vi "HostoldMain.vi"() -> ()   [LabVIEW 2009]
uses:
  <vilib>/rvi/interface/nirviOpenFPGA/nirviOpenFPGA.xnode
  <vilib>/rvi/interface/nirviReadWriteControl/nirviReadWriteControl.xnode
  <vilib>/rvi/interface/nirviCloseFPGA/nirviCloseFPGA.xnode
  States.ctl
  <vilib>/rvi/interface/nirviMethod/nirviMethod.xnode
  Pulse Acquisition/5122-States.ctl
  <instrlib>/niScope/Configure/Trigger/niScope Configure Trigger Edge.vi
  <instrlib>/niScope/Acquire/Fetch/niScope Fetch.vi
  <vilib>/Analysis/NI_AALPro.lvlib
  <vilib>/Utility/file.llb/Write To Spreadsheet File (DBL).vi
  B Field control Signal/B-Generator States.ctl
  <vilib>/DAQmx/create/channels.llb/DAQmx Create Channel (AO-Voltage-Basic).vi
  <vilib>/DAQmx/configure/timing.llb/DAQmx Timing (Sample Clock).vi
  <vilib>/DAQmx/configure/trigger.llb/DAQmx Start Trigger (Digital Edge).vi
  Program Files (x86)/National Instruments/LabVIEW 2009/resource/objmgr/daqmx.rc
  <vilib>/DAQmx/write.llb/DAQmx Write (Analog 1D DBL 1Chan NSamp).vi
  <vilib>/Utility/error.llb/DialogType.ctl
  FPGA Bitfiles/MOT2.lvproj_FPGA Target_FPGAvi.vi.lvbitx
  Signal Options.ctl
  FPGAvi.vi
  Sequence.ctl
  <instrlib>/Agilent ESG Series/Agilent ESG Series.lvlib
  Raman Measure/Raman.ctl
  <vilib>/DAQmx/create/channels.llb/DAQmx Create Channel (AI-Voltage-Basic).vi
  <vilib>/DAQmx/read.llb/DAQmx Read.vi
  <vilib>/DAQmx/read.llb/DAQmx Read (Analog 2D DBL NChan NSamp).vi
  <vilib>/Analysis/NI_AALBase.lvlib
  <vilib>/userDefined/High Color/nirio_resource_hc.ctl
  <instrlib>/niScope/Controls/niScope vertical coupling.ctl
panel:
  out "data":dbl[][](array[numeric]) format="%0.6f"
  in  "Output  Trigger Sign (DIO1)":bool
  in  "Signal Trigger Source (DIO0)":bool=TRUE
  in  "Pulse Selection":bool
  in  "Switch Chopper \nWindow Trigger":bool
  in  "Master Stop":bool
  in  "Tab Control":T1(tab)
  out "Acquisition Rate":dbl[unit]=0.02 min=0.0 max=107374.18239999999
  in  "Pulse Repetition Period":dbl[unit]=0.02
  out "Memory Sequence Duration":dbl[unit]=0.02 min=0.0 max=107374.18239999999
  out "Chopper 1/2 Dark Time":dbl[unit]
  in  "DLCZ Period":dbl[unit]=1e-06
  in  "DLCZ Pulse Duration":dbl[unit]=5.0000000000000004e-08
  in  "DLCZ Stop":dbl[unit]=0.004 caption="Stop"
  in  "DLCZ Start":dbl[unit] caption="Start"
  in  "B-Field Extinction Time":dbl[unit]=0.00125 min=0.0 max=107374.18239999999
  in  "Min. Measurement Period":dbl[unit]=0.02 caption="Meas. Period" min=0.0 max=107374.18239999999
  in  "Opt Density Delay (DIO7)":dbl[unit]
  in  "Opt Density Duration (DIO7)":dbl[unit]=0.000125
  in  "Signal Delay (DIO6)":dbl[unit]
  in  "Signal Duration (DIO6)":dbl[unit]=0.000125
  in  "Control Delay(DIO5/1)":dbl[unit] min=0.0 max=107374.18239999999
  in  "Control Duration (DIO5/1)":dbl[unit]=0.000125 min=0.0 max=107374.18239999999
  in  "FPGA Target":T2="FPGA"
  out "Active":bool
  in  "Memory Mode":T3=enum."Generate DLCZ Pulses"
  in  "Trapping (DIO3)":dbl[unit]=0.0015 min=0.0 max=107374.18239999999
  in  "Repump (DIO4)":dbl[unit]=0.0015
  in  "Pump (DIO8)":dbl[unit]=0.0015
  out "Graphing":bool
  out "Generated Signals":digitalwaveform(graph)
  in  "Activate Raman Acquisition":bool=TRUE
  in  "Scan Frequency":bool
  out "Acquisition Count":i32
  in  "Number of Measurements":u32=10
  in  "Samples per Channel":i32=2048 caption="Measurement Samples"
  in  "VISA session":refnum<visa-resource-name>="GPIB0::19::INSTR"
  out "Current Frequency":dbl[unit]
  in  "Start Frequency":dbl[unit]=-5000000.0
  in  "Stop Frequency":dbl[unit]=5000000.0
  in  "Resonance Frequency":dbl[unit]=100000000.0
  in  "Upper Threshold (% of Max)":dbl=80.0
  in  "Lower Threshold (% of Min)":dbl=120.0
  in  "Number of Frequency Intervals":u32=100
  out "Frequency Interval":dbl[unit]
  in  "Raman Measurement File":path=path "C:/Users/atomes/Desktop/Labview Projects/MOT2/raman.txt"
  out "Measurement":dbl[][](graph) caption="Pulse Monitor"
  out "Raman Measure":cluster{dbl[], dbl[]}[](graph)
  in  "Ramand Control Duration (DIO5)":dbl[unit]=0.000125 min=0.0 max=107374.18239999999
  in  "Raman Control Delay(DIO5)":dbl[unit] min=0.0 max=107374.18239999999
  in  "Raman Signal Delay (DIO6)":dbl[unit]
  in  "Raman Signal Duration (DIO6)":dbl[unit]=0.000125
  in  "Acquisition Delay":dbl[unit] format="%.2f"
  out "Interval Between Samples":dbl[unit]
  out "Actual Sample Rate":dbl[unit]
  in  "Desired Sample Rate":dbl[unit]=100000000.0 caption="Min. Sample Rate" step=1.0 format="%.2p"
  in  "Acquisition Time per Pulse":dbl[unit]=0.0005 format="%#.2g"
  out "Acquisitions Remaining":i32 caption="Number of Runs"
  in  "Data Output":path=path "F:/data/test.txt"
  in  "Number of Pulses to Record":i32=1 caption="Number of Runs" format="%.0p"
  out "Total Acquired Time":dbl[unit]
  out "Total Number of Datapoints":i32=1000000
  out "Total Experiment Time":dbl[unit]
  out "Number of Samples per Pulse":i32
  in  "Vertical range (0 to 10V)":dbl[unit]=4.0 caption="Vertical Range (V)" format="%.2f"
  in  "Vertical coupling":T4=1 caption="Vertical Coupling" items=["AC", "DC", "Ground"]
  in  "Channel":u16(ring) items=["0", "1"]
  out "Acquisition Sequence":dbl[][](graph)
  in  "Get Reference Parameters":bool
  in  "Capture":bool
  in  "Acquire Data":bool
  out "Global EIT Delay":dbl[unit] format="%#.2g"
  out "Risetime Chart":cluster{dbl}(graph)
  out "Falltime Chart":cluster{dbl}(graph)
  out "Width Chart":cluster{dbl}(graph)
  out "Delay Chart":cluster{dbl}(graph)
  out "Amplitude Chart":cluster{dbl}(graph)
  out "Risetime":string
  out "Falltime":string
  out "Pulse Width":string
  out "Delay":string
  out "Amplitude":string
  out "Memory Duration":dbl[unit]
  in  "Global Delay":dbl[unit]=3e-06
  in  "High Voltage (V Hi)":dbl[unit]=5.0
  in  "Trigger Control":bool=TRUE
  in  "Activate B-Field":bool=TRUE
  out "B-Field Control Signal":dbl[](graph)
  in  "V4":dbl[unit]
  in  "V3":dbl[unit]
  in  "V2":dbl[unit]=-5.0
  in  "V1":dbl[unit]=-5.0 min=-10.0 max=10.0
  in  "B":dbl[unit]=0.003
  in  "A":dbl[unit]=9.999999999999999e-05
  out "t_last_chop+t_dark-t_off":dbl[unit]
  out "Current State":T5
  out "Cut Initiated":dbl[unit]
  out "B-Field Extinction Time 2":dbl[unit]
  out "Memory Mode 2":T3=enum."Coherent Memory Sequence"
  in  "Epsilon":dbl[unit]
  out "Memory Timer":dbl[unit]
  out "Global Time":dbl[unit]
  out "t_chop":dbl[unit]
  out "T_last-chop + t_dark":dbl[unit]
  out "Last DLCZ Period":dbl[unit]
  out "Reference Pulse":dbl[](array[numeric])
  out "Channel String":string
  # "Chopper"
  # "Internal"
  # "All Pulses"
  # "1 out of 2 Pulses"
  # "Delays"
  # "Durations"
  # "Chopper Measurement and MOT Timing"
  # "DLCZ Pulse Train (DIO5)"
  # "Width"
  # "Period"
  # "Optical Density (DIO7)"
  # "Signal (DIO6)"
  # "Control  (DIO5)"
  # "Extinction Time"
  # "Delays"
  # "Durations"
  # "Raman Signal (DIO6)"
  # "Raman Control (DIO5)"
  # "Optical Pulse Acquisition"
  # "Pulse Statistics"
  # "Trigger must be sent \nto begin generation"
  # "Example Diagram"
  # "Voltages"
  # "Intervals"
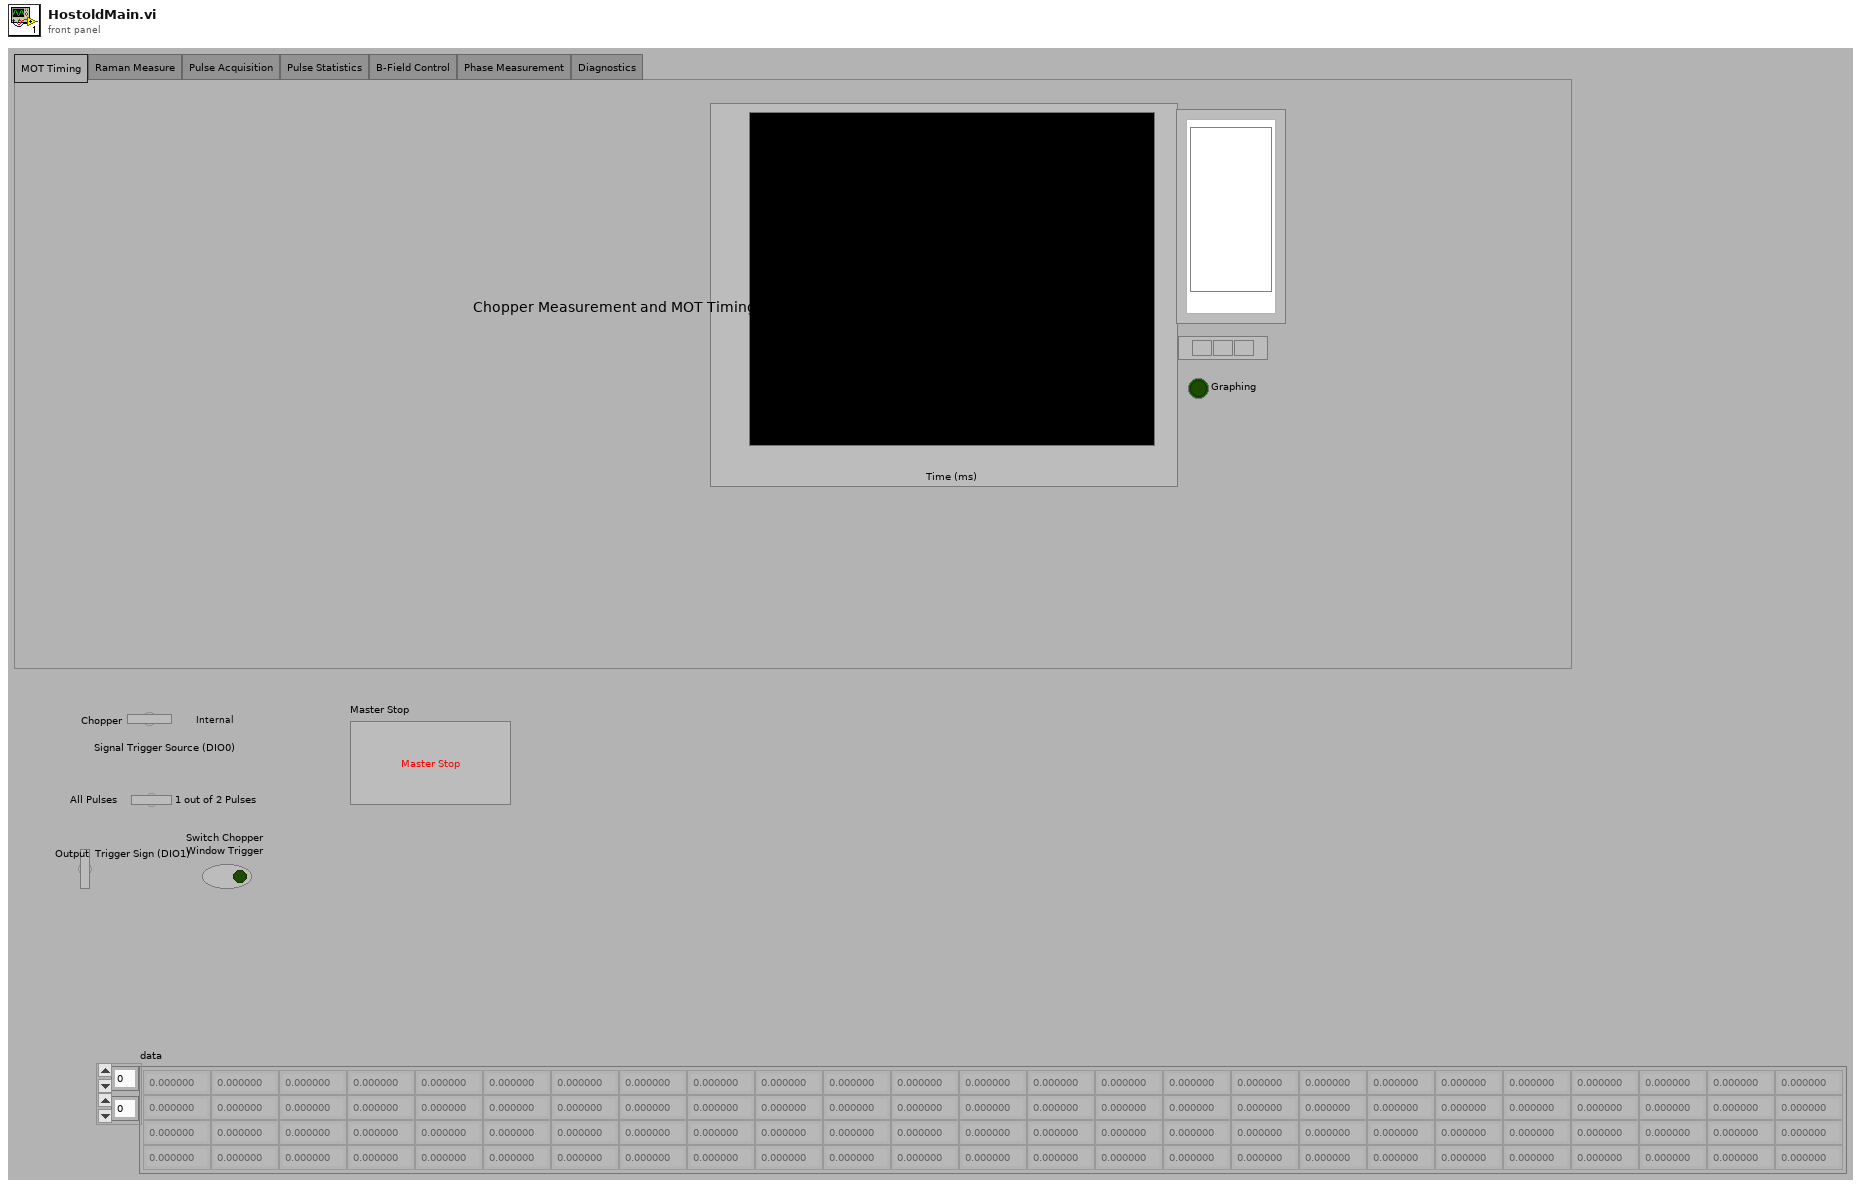
[diagram p1: front panel]
types:
  T1 = enum32{"MOT Timing", "Raman Measure", "Pulse Acquisition", "Pulse Statistics", "B-Field Control", "Phase Measurement", "Diagnostics"}
  T2 = typedef "nirio_resource_hc.ctl" = tag
  T3 = typedef "Signal Options.ctl" = enum16{"Cycle Trap - Standby", "Generate DLCZ Pulses", "Measure Optical Density", "Measure Raman", "Single Photon Memory Efficiency", "Coherent Memory Sequence", "Squeezed AOM Memory Sequence", "Squeezed Chopper Memory Sequence"}
  T4 = typedef "niScope vertical coupling.ctl" = i32
  T5 = typedef "Sequence.ctl" = enum16{"Build MOT", "Memory Sequence", "Alignment - Lights On"}
  T6 = typedef "Raman.ctl" = enum16{"Initialize", "Monitor Pulses", "Stop Raman Acquisition", "Scan Frequency", "Output Data", "Standby"}
  T7 = typedef "States.ctl" = enum16{"Initialize", "Send Data", "Receive Data", "Update Graph", "Check for Activity", "Close"}
  T8 = typedef "DialogType.ctl" = u16
  T9 = typedef "B-Generator States.ctl" = enum16{"Initialize", "Start Task", "Check Task", "Stop Task", "Stop"}
  T10 = typedef "5122-States.ctl" = enum16{"Initialize Card", "Continuous Mode", "Fetch", "Snapshot Acquistion", "Standby", "Record DataFile", "Exit"}
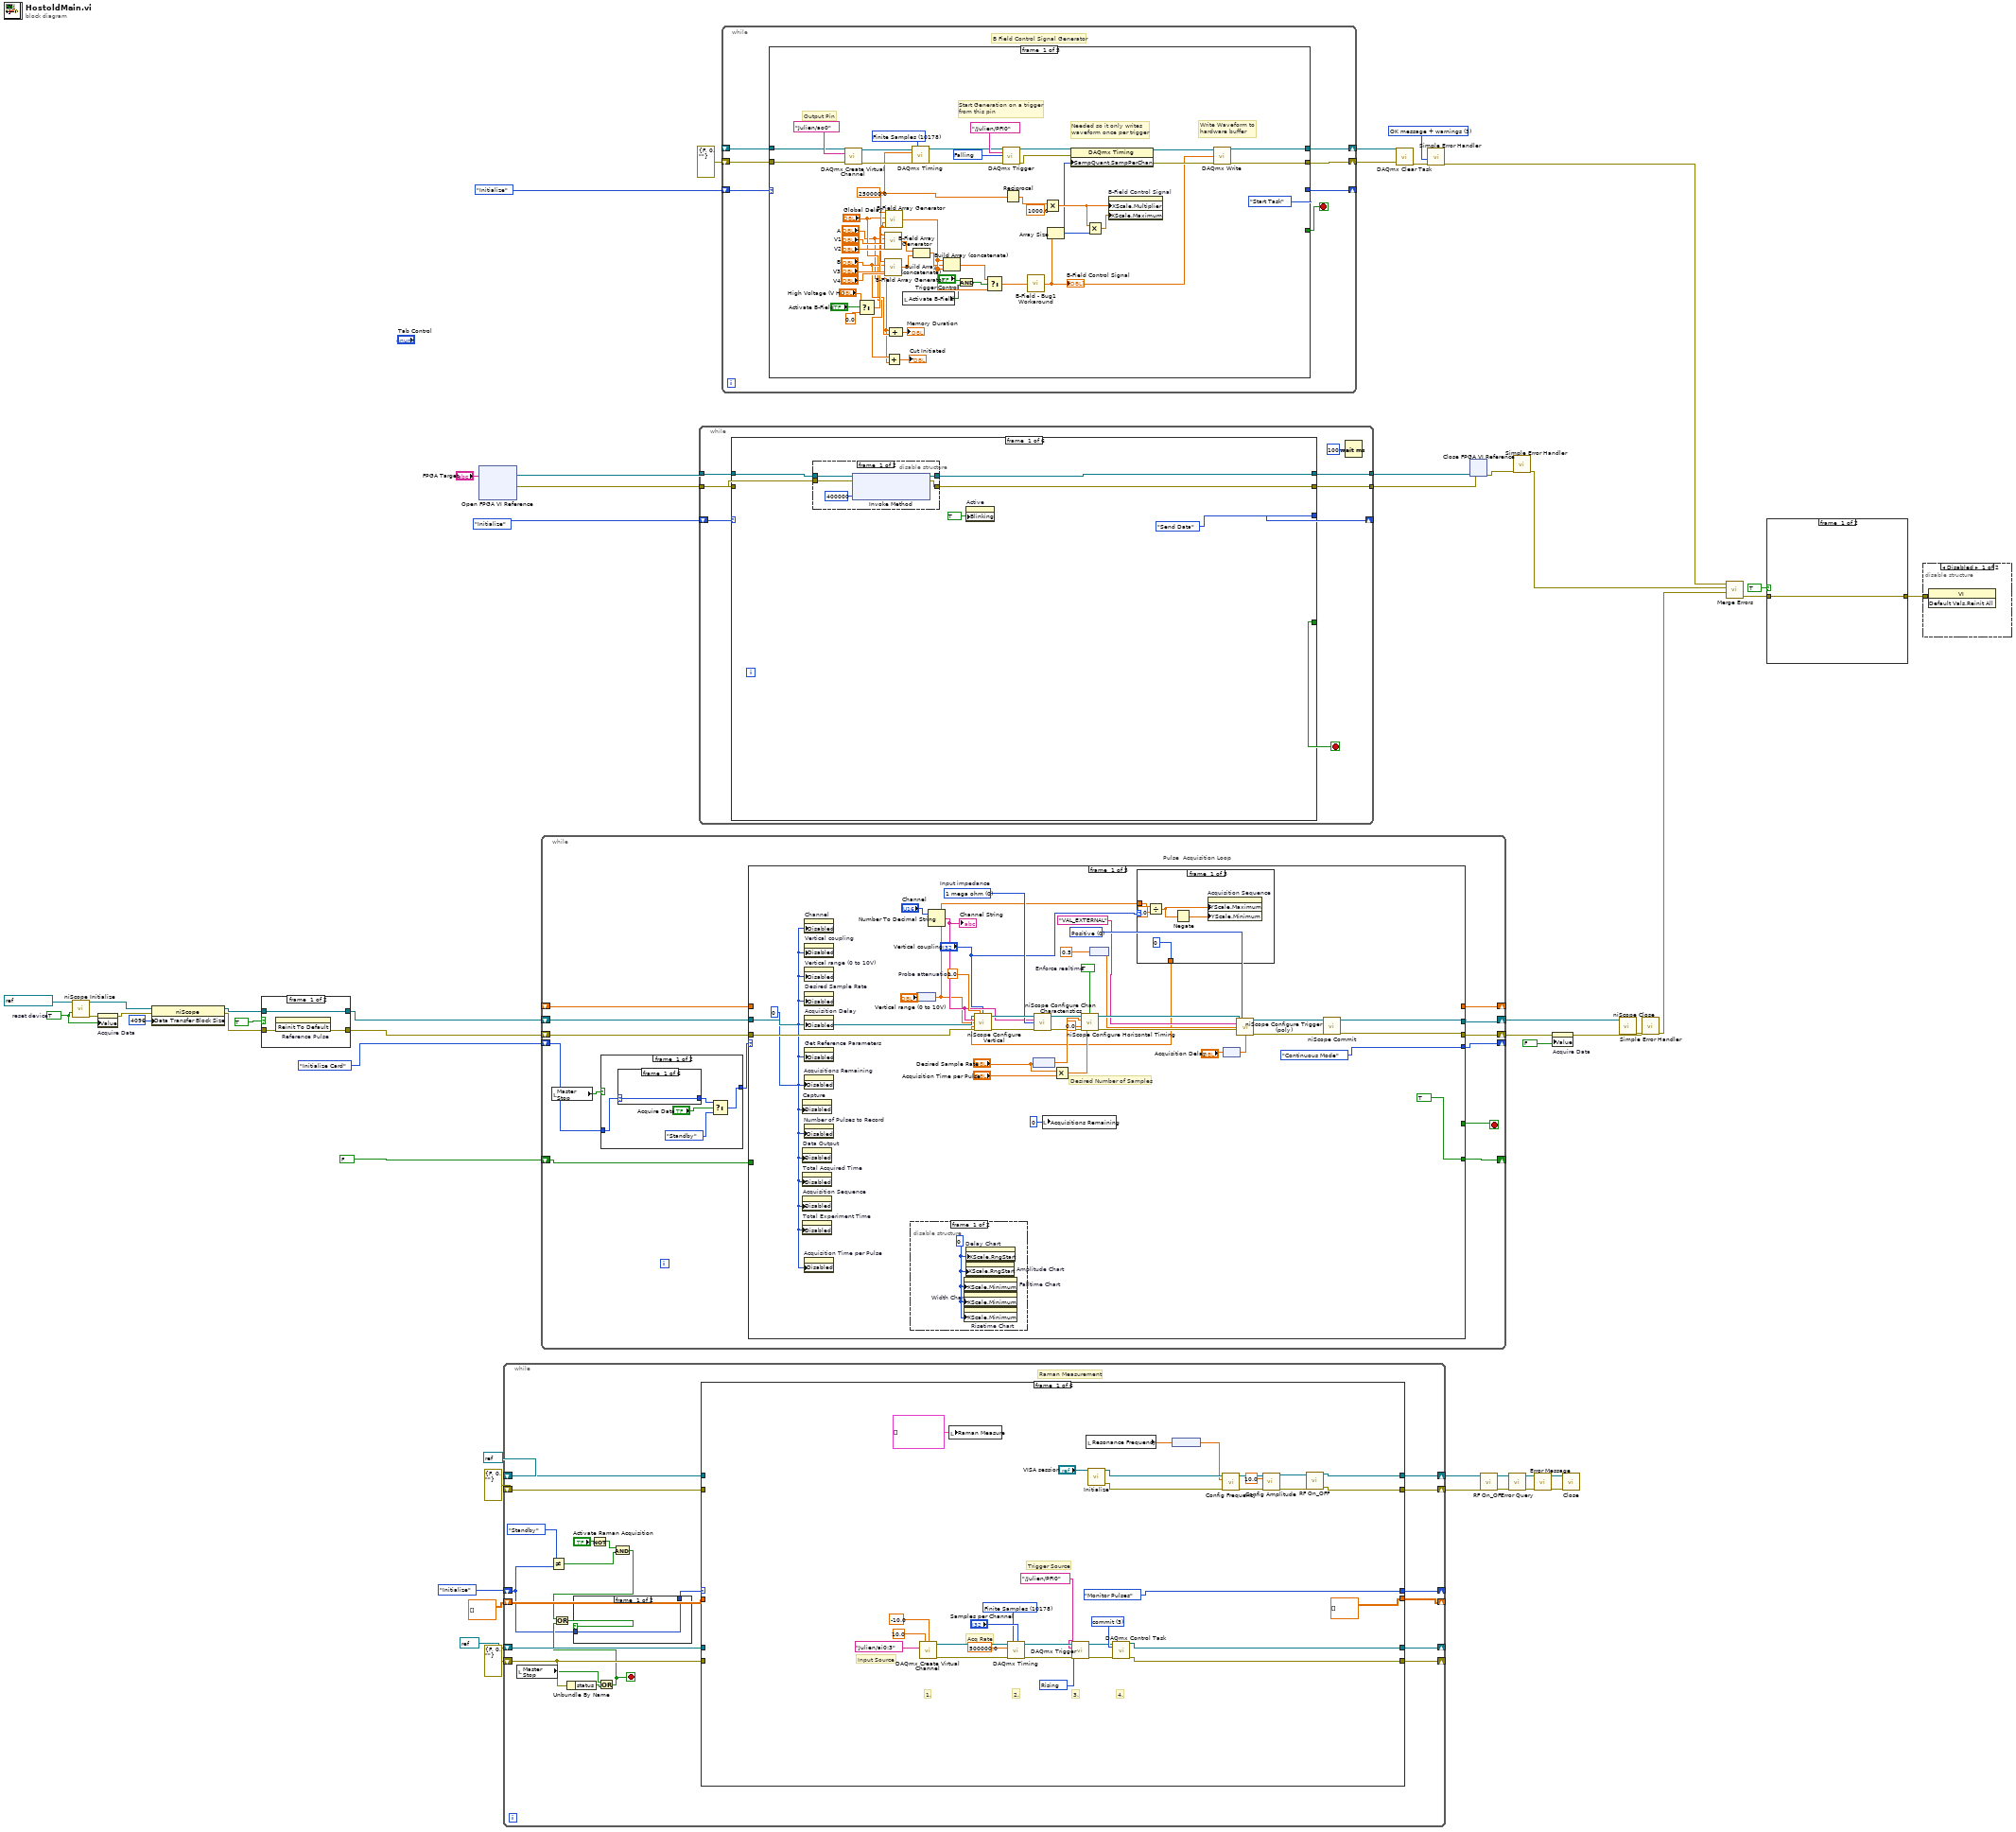
[diagram p0: block diagram]
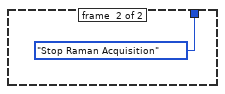
[diagram p2: hidden frame]
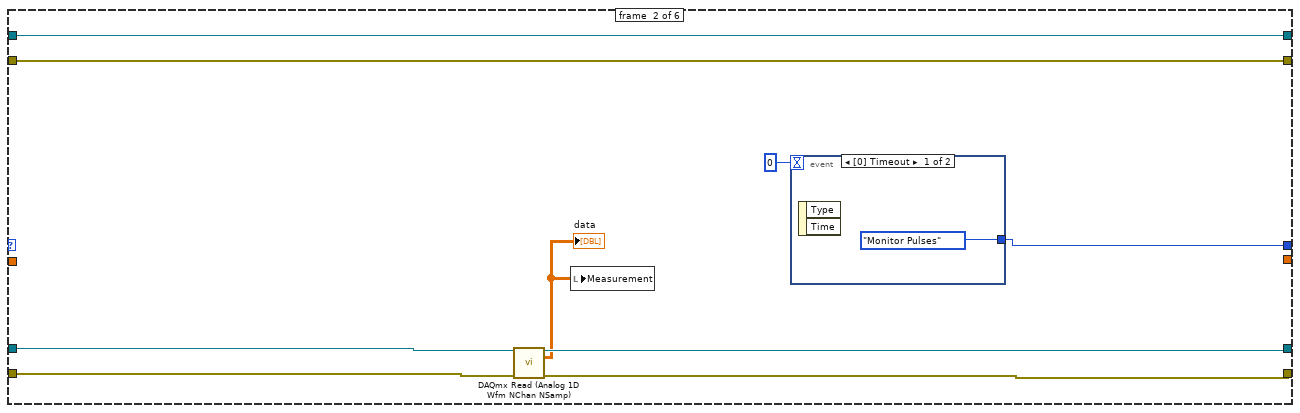
[diagram p3: hidden frame]
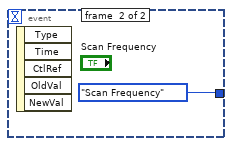
[diagram p4: hidden frame]
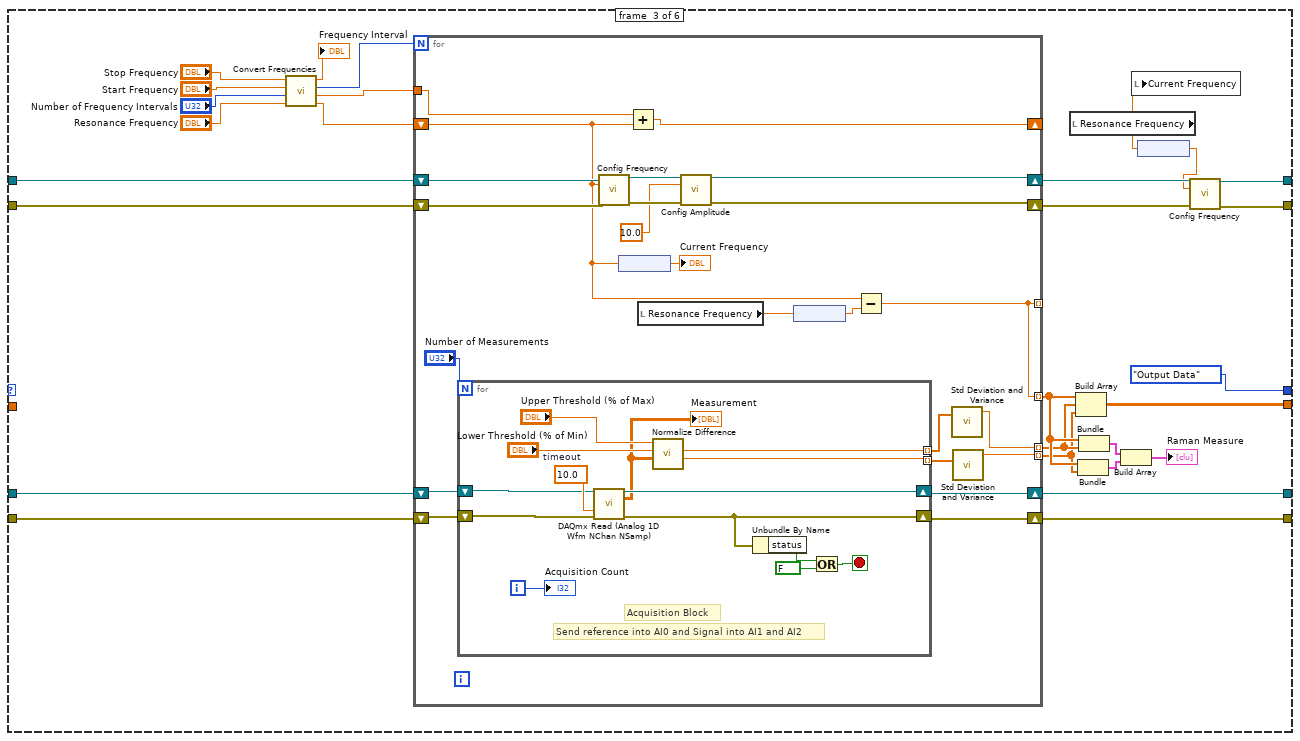
[diagram p5: hidden frame]
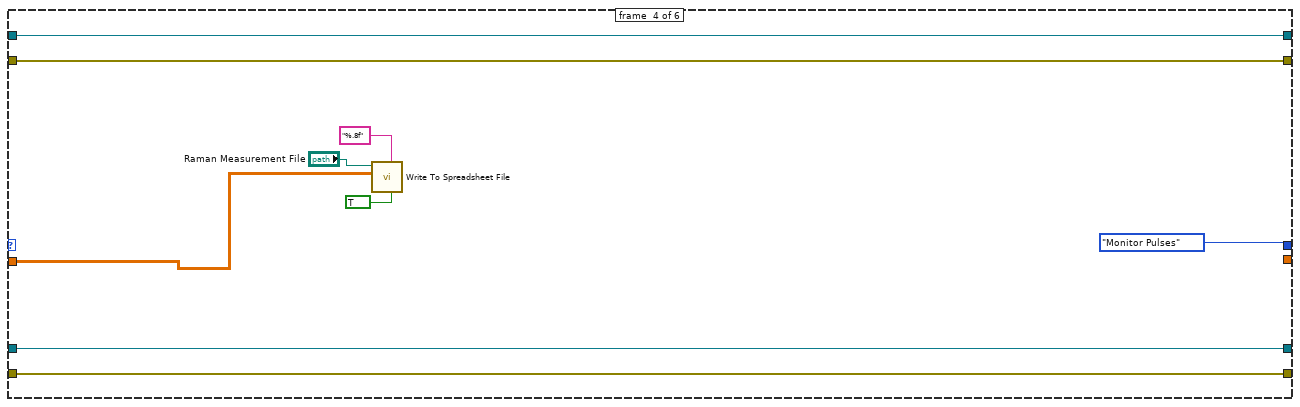
[diagram p6: hidden frame]
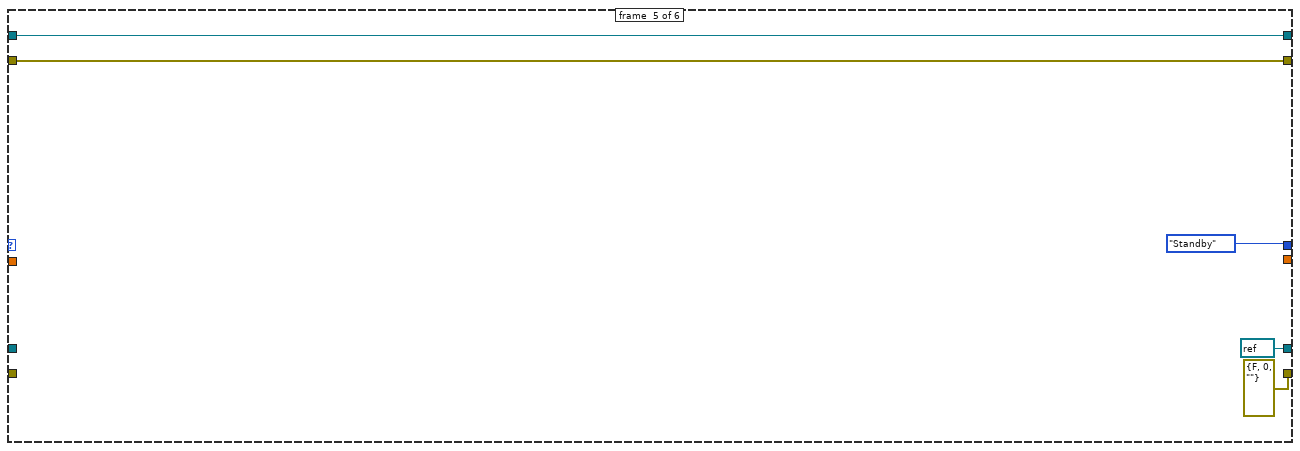
[diagram p7: hidden frame]
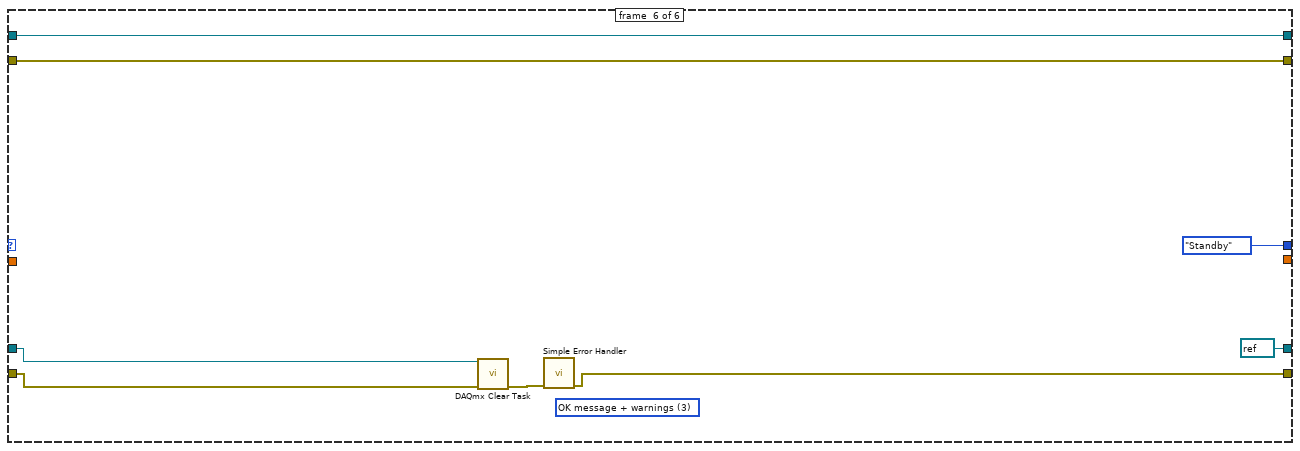
[diagram p8: hidden frame]
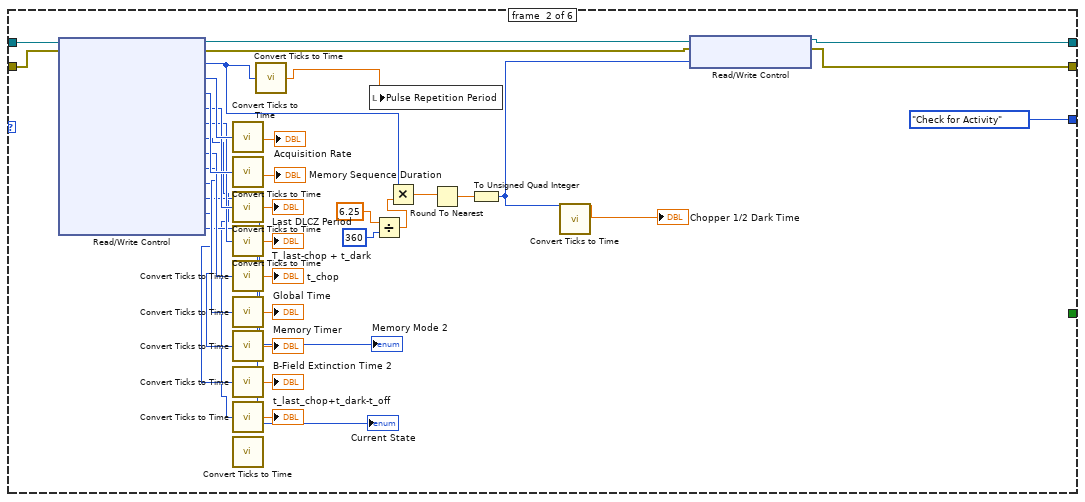
[diagram p10: hidden frame]
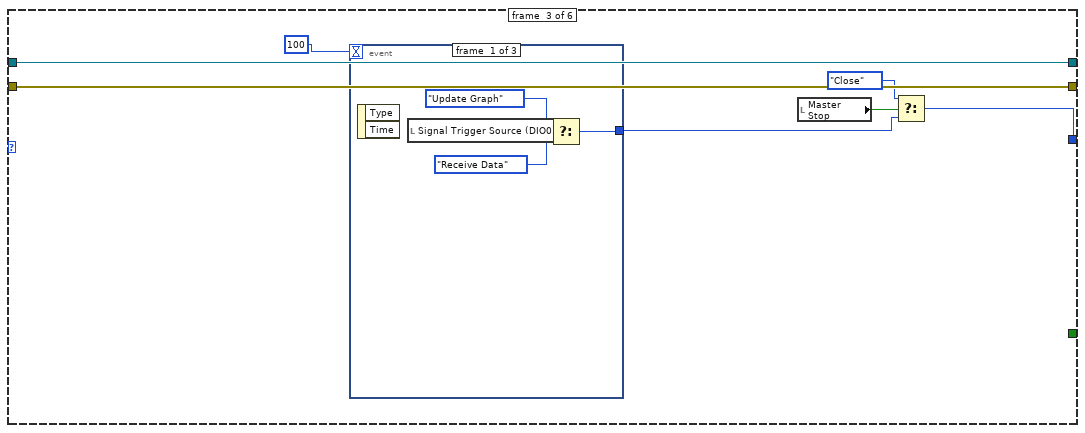
[diagram p11: hidden frame]
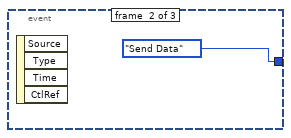
[diagram p12: hidden frame]
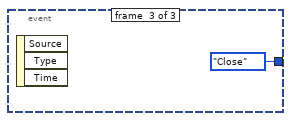
[diagram p13: hidden frame]
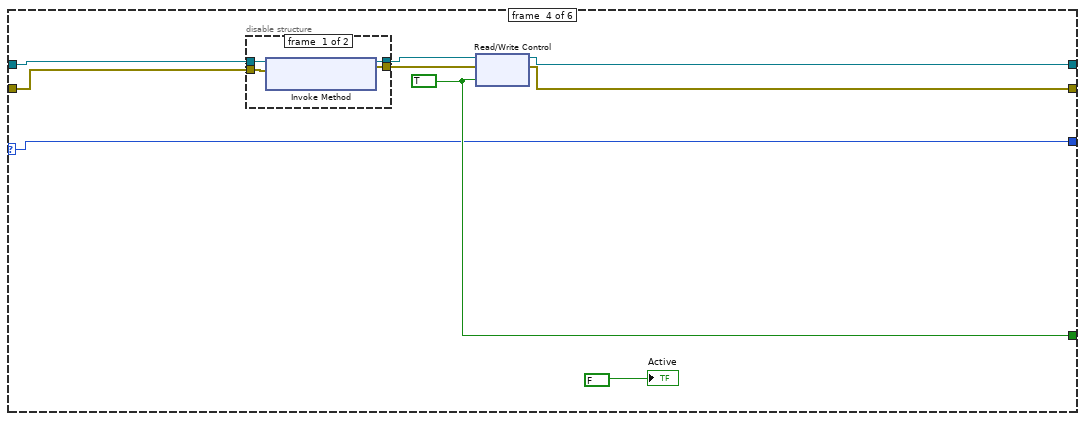
[diagram p14: hidden frame]
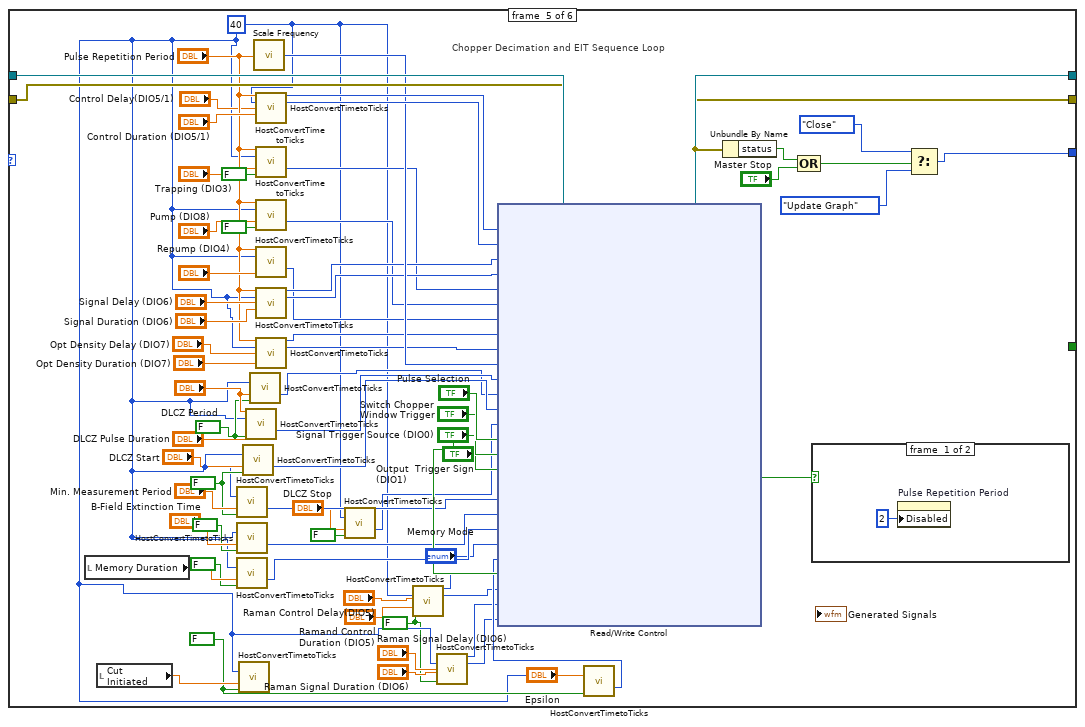
[diagram p16: hidden frame]
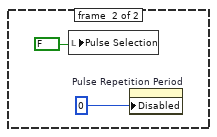
[diagram p17: hidden frame]
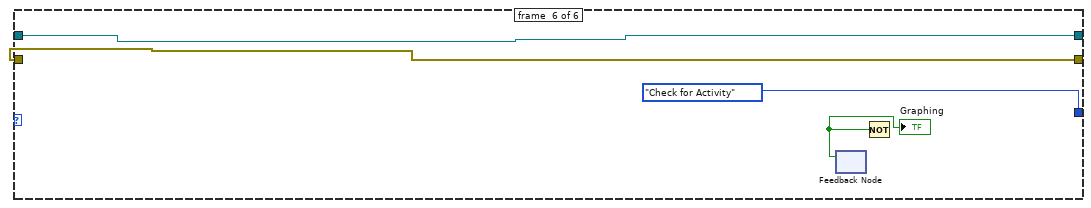
[diagram p18: hidden frame]
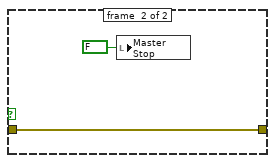
[diagram p20: hidden frame]
diagram:
  w33 = T8 3 items=["no dialog", "OK message", "continue or stop message", "OK message + warnings", "continue/stop + warnings"] ("type of dialog (OK msg:1)")
  w44 = TRUE  # reset device
  n1 = call <instrlib>:"niScope Initialize.vi"("resource name"=refnum<k15> "Acquisition" ("Resource name 5"), "reset device"=w44) -> ("instrument handle"=w48:refnum<k15>, "error out"=w46:errorcluster)  [unwired: 2 in, 10 out]
  n2 = property on="Acquire Data" class="Bool (strict)"(error in=w46, "Value"=w44) -> (error out=w45:errorcluster)  [unwired: 1 in, 1 out]
  n3 = property class="niScope"(reference=w48, error in=w45, "Data Transfer Block Size"=4096) -> (reference out=w38:refnum<k15>, error out=w36:errorcluster)
  n4 = case shown="True" TRUE {
    tunnel: [w53 w55] -> w37
    tunnel: w38 -> [w53 w55]
    tunnel: [w52 w54] -> w35
    tunnel: w36 -> [w52 w54]
    frame #0 {
      n5 = invoke on="Reference Pulse" class="Arr (strict)" method="Reinit To Default"() -> ()  [unwired: 3 in, 3 out]
    }
    frame #1 {
    }
  }
  n6 = xnode "Open FPGA VI Reference"("resource name"="FPGA Target") -> ("FPGA VI Reference Out"=w17:refnum<k20>, "error out"=w15:errorcluster)  [unwired: 1 in]
  n7 = while {
    shift-right: [w73] -> _
    shift-left: Raman."Initialize" ("Raman State") -> [w59]
    shift-right: [w76] -> _
    shift-left: refnum<k21> refnum ("task out") -> [w72]
    shift-right: [w77] -> _
    shift-left: errorcluster {"status"=FALSE, "code"=0, "source"=""} ("error out") -> [w66]
    shift-right: [w68] -> _
    shift-left: dbl[][] [] -> [w71]
    shift-right: [w74] -> w14
    shift-left: refnum<visa-resource-name> refnum ("VISA Resource Name Out") -> [w70]
    shift-right: [w75] -> w6
    shift-left: errorcluster {"status"=FALSE, "code"=0, "source"=""} ("error out") -> [w69]
    stop <- w63 stop-if-true
    # "Raman Measurement"
    n8 = local read "Master Stop"() -> (w64:bool)
    n9 = Not Equal?(x=Raman."Standby" ("Raman State"), y=w59) -> (x != y?=w57:bool)
    n10 = Unbundle By Name(w66) -> ("status"=w65:bool)
    n11 = Not(x="Activate Raman Acquisition") -> (.not. x?=w60:bool)
    n12 = Or(x=w64, y=w65) -> (x .or. y?=w63:bool)
    n13 = And(x=w60, y=w57) -> (x .and. y?=w56:bool)
    n14 = Or(x=w56, y=w63) -> (x .or. y?=w62:bool)
    n15 = case shown="False" w62 {
      tunnel: [w78 Raman."Stop Raman Acquisition" ("Raman State")] -> w61
      tunnel: w59 -> [w78 _]
      frame #0 {
      }
      frame #1 {
      }
    }
    n16 = case shown="\"Monitor Pulses\"" w61 {
      tunnel: [w95 w114 w150 w190 errorcluster {"status"=FALSE, "code"=0, "source"=""} ("error out") w203] -> w77
      tunnel: [w96 w115 w149 w191 refnum<k21> refnum ("task out") refnum<k21> refnum ("task out")] -> w76
      tunnel: [w83 w119 w135 w188 w200 w207] -> w75
      tunnel: [w82 w120 w136 w189 w201 w208] -> w74
      tunnel: [Raman."Monitor Pulses" ("Raman State") w112 Raman."Output Data" ("Raman State") Raman."Monitor Pulses" ("Raman State") Raman."Standby" ("Raman State") Raman."Standby" ("Raman State")] -> w73
      tunnel: w72 -> [_ w117 w142 w191 _ w205]
      tunnel: w66 -> [_ w116 w141 w190 _ w204]
      tunnel: w71 -> [_ _ _ w194 _ _]
      tunnel: w70 -> [_ w120 w139 w189 w201 w208]
      tunnel: w69 -> [_ w119 w138 w188 w200 w207]
      tunnel: [dbl[][] [] ("Frequency/Delta Pairs") _ w124 _ _ _] -> w68
      frame #0 {
        w111 = 10280 items=["Rising"=10280, "Falling"=10171] ("edge")
        w102 = 3 items=["verify"=2, "reserve"=4, "commit"=3, "unreserve"=5, "abort"=6] ("action")
        w103 = 10178 items=["Finite Samples"=10178, "Continuous Samples"=10123] ("sample mode")
        # "Input Source"
        # "Acq Rate"
        # "Trigger Source"
        # "4."
        # "3."
        # "2."
        # "1."
        n17 = call-poly <vilib>:"DAQmx Create Virtual Channel.vi"("maximum value"=10.0 ("Maximum Value"), "minimum value"=-10.0 ("Minimum Value"), "physical channels"=tag "Julien/ai0:3" ("Physical Channel")) -> ("task out"=w105:refnum<k21>, "error out"=w108:errorcluster)  [unwired: 11 in]
        n18 = local write "Raman Measure"(cluster{dbl[], dbl[]}[] [] ("Raman Measure")) -> ()
        n19 = call-poly <vilib>:"DAQmx Timing.vi"("task/channels in"=w105, "sample mode"=w103, "samples per channel"="Samples per Channel", "rate"=500000.0 ("Rate"), "error in"=w108) -> ("task out"=w101:refnum<k21>, "error out"=w100:errorcluster)  [unwired: 9 in]
        n20 = call-poly <vilib>:"DAQmx Trigger.vi"("task/channels in"=w101, "source"=tag "/Julien/PFI0" ("Trigger source"), "edge"=w111, "error in"=w100) -> ("task out"=w99:refnum<k21>, "error out"=w98:errorcluster)  [unwired: 10 in]
        n21 = local read "Resonance Frequency"() -> (w90:dbl[unit])
        n22 = call <instrlib>:"Initialize.vi"("VISA Resource Name"="VISA session") -> ("VISA Resource Name Out"=w92:refnum<visa-resource-name>, "error out"=w91:errorcluster)  [unwired: 4 in, 9 out]
        n23 = call <vilib>:"DAQmx Control Task.vi"("task/channels in"=w99, "action"=w102, "error in"=w98) -> ("task out"=w96:refnum<k21>, "error out"=w95:errorcluster)  [unwired: 11 in]
        n24 = node(w90) -> (w89:dbl)
        n25 = call <instrlib>:"Config Frequency.vi"("VISA Resource Name"=w92, "Frequency (1000.0)"=w89, "error in (no error)"=w91) -> ("VISA Resource Name Out"=w88:refnum<visa-resource-name>, "error out"=w87:errorcluster)  [unwired: 6 in, 5 out]
        n26 = call <instrlib>:"Config Amplitude.vi"("VISA Resource Name"=w88, "Amplitude (-135.00)"=10.0, "error in (no error)"=w87) -> ("VISA Resource Name Out"=w85:refnum<visa-resource-name>, "error out"=w84:errorcluster)  [unwired: 5 in, 6 out]
        n27 = call <instrlib>:"RF On_OFF.vi"("VISA Resource Name"=w85, "error in (no error)"=w84) -> ("VISA Resource Name Out"=w82:refnum<visa-resource-name>, "error out"=w83:errorcluster)  [unwired: 1 in, 11 out]
      }
      frame #1 {
        n28 = call-poly "DAQmx Read (Analog 1D Wfm NChan NSamp).vi"("task/channels in"=w117, "error in"=w116) -> ("task out"=w115:refnum<k21>, "data"=w113:dbl[][], "error out"=w114:errorcluster)  [unwired: 11 in]
        "data" <- w113
        n29 = local write "Measurement"(w113) -> ()
        n30 = event shown="[0] Timeout" {
          selector: _ -> [_ _]
          dyn-events: _ -> [_ _]
          timeout: 0 -> [_ _]
          tunnel: [Raman."Monitor Pulses" ("Raman State") Raman."Scan Frequency" ("Raman State")] -> w112
          event #0 {
            n31 = event-data() -> ()  [unwired: 1 in, 2 out]
          }
          event #1 {
            n32 = event-data() -> ()  [unwired: 1 in, 5 out]
          }
        }
      }
      frame #2 {
        n33 = call "Convert Frequencies.vi"("Resonance Frequency (MHz)"="Resonance Frequency", "Number of Intervals"="Number of Frequency Intervals", "Start Frequency (MHz)"="Start Frequency", "Stop Frequency (MHz)"="Stop Frequency") -> ("Start Frequency (Number)"=w144:dbl, "Frequency Increment (Number)"=w145:dbl, "Number of Intervals (Out)"=w146:u32, "Frequency Interval"=→"Frequency Interval":dbl[unit])
        n34 = for {
          N: w146 -> [_]
          shift-right: [w172] -> w149
          shift-left: w142 -> [w170]
          shift-right: [w173] -> w150
          shift-left: w141 -> [w171]
          tunnel: w145 -> [w167]
          shift-right: [w161] -> _
          shift-left: w144 -> [w152]
          shift-right: [w163] -> w137
          shift-left: w139 -> [w166]
          shift-right: [w162] -> w134
          shift-left: w138 -> [w165]
          tunnel: [w164] -> w126 mode=indexing
          tunnel: [w153] -> w127 mode=indexing
          tunnel: [w156] -> w125 mode=indexing
          tunnel: [w153] -> _ mode=indexing
          n35 = for {
            N: "Number of Measurements" -> [_]
            shift-right: [w178] -> w172
            shift-left: w170 -> [w180]
            shift-right: [w177] -> w173
            shift-left: w171 -> [w179]
            tunnel: [w183] -> w168 mode=indexing
            tunnel: [w182] -> w157 mode=indexing
            i -> [w184]
            stop <- w185 stop-if-true
            w187 = 10.0  # timeout
            # "Acquisition Block"
            # "Send reference into AI0 and Signal into AI1 and AI2"
            n36 = call-poly "DAQmx Read (Analog 1D Wfm NChan NSamp).vi"("task/channels in"=w180, "timeout"=w187, "error in"=w179) -> ("task out"=w178:refnum<k21>, "data"=w174:dbl[][], "error out"=w177:errorcluster)  [unwired: 10 in]
            "Measurement" <- w174
            n37 = call "Normalize Difference.vi"("data"=w174, "Lower Threshold (% of Min)"="Lower Threshold (% of Min)", "Upper Threshold (% of Max)"="Upper Threshold (% of Max)") -> ("Normalized Difference (Reference - Signal 2)"=w182:dbl, "Normalized Difference  (Reference - Signal1)"=w183:dbl)  [unwired: 6 in, 1 out]
            n38 = Unbundle By Name(w177) -> ("status"=w186:bool)
            n39 = Or(x=w186, y=FALSE) -> (x .or. y?=w185:bool)
            "Acquisition Count" <- w184
          }
          n40 = call <instrlib>:"Config Frequency.vi"("VISA Resource Name"=w166, "Frequency (1000.0)"=w152, "error in (no error)"=w165) -> ("VISA Resource Name Out"=w159:refnum<visa-resource-name>, "error out"=w160:errorcluster)  [unwired: 6 in, 5 out]
          n41 = node(w152) -> (→"Current Frequency":dbl[unit])
          n42 = Add(x=w167, y=w152) -> (x+y=w161:dbl)
          n43 = local read "Resonance Frequency"() -> (w155:dbl[unit])
          n44 = call <instrlib>:"Config Amplitude.vi"("VISA Resource Name"=w159, "Amplitude (-135.00)"=10.0, "error in (no error)"=w160) -> ("VISA Resource Name Out"=w163:refnum<visa-resource-name>, "error out"=w162:errorcluster)  [unwired: 5 in, 6 out]
          n45 = node(w155) -> (w154:dbl)
          n46 = Subtract(x=w152, y=w154) -> (x-y=w153:dbl)
          n47 = call <vilib>:"Std Deviation and Variance.vi"("X"=w168) -> ("mean"=w164:dbl)  [unwired: 1 in, 2 out]
          n48 = call <vilib>:"Std Deviation and Variance.vi"("X"=w157) -> ("mean"=w156:dbl)  [unwired: 1 in, 2 out]
        }
        n49 = local read "Resonance Frequency"() -> (w123:dbl[unit])
        n50 = Build Array(w127, w126, w125) -> (w124:dbl[][])
        n51 = Bundle(w127, w125) -> (w129:cluster{dbl[], dbl[]})  [unwired: 1 in]
        n52 = Bundle(w127, w126) -> (w130:cluster{dbl[], dbl[]})  [unwired: 1 in]
        n53 = Build Array(w130, w129) -> (→"Raman Measure":cluster{dbl[], dbl[]}[])
        n54 = local write "Current Frequency"(w123) -> ()
        n55 = node(w123) -> (w133:dbl)
        n56 = call <instrlib>:"Config Frequency.vi"("VISA Resource Name"=w137, "Frequency (1000.0)"=w133, "error in (no error)"=w134) -> ("VISA Resource Name Out"=w136:refnum<visa-resource-name>, "error out"=w135:errorcluster)  [unwired: 6 in, 5 out]
      }
      frame #3 {
        n57 = call-poly <vilib>:"Write To Spreadsheet File.vi"("transpose? (no:F)"=TRUE, "format (%.3f)"="%.8f", "2D data"=w194, "file path (dialog if empty)"="Raman Measurement File") -> ()  [unwired: 4 in, 1 out]
      }
      frame #4 {
      }
      frame #5 {
        (unwired) T8 3 items=["no dialog", "OK message", "continue or stop message", "OK message + warnings", "continue/stop + warnings"] ("type of dialog (OK msg:1)")
        n58 = call <vilib>:"DAQmx Clear Task.vi"("task in"=w205, "error in"=w204) -> ("error out"=w206:errorcluster)  [unwired: 13 in]
        n59 = call <vilib>:"Simple Error Handler.vi"("error in (no error)"=w206) -> ("error out"=w203:errorcluster)  [unwired: 4 in, 4 out]
      }
    }
  }
  n60 = while {
    shift-right: [w215] -> _
    shift-left: 5122-States."Initialize Card" ("Enum") -> [w213]
    shift-right: [w222] -> w50
    shift-left: w37 -> [w220]
    shift-right: [w221] -> w43
    shift-left: w35 -> [w219]
    shift-right: [w218] -> _
    shift-left: _ -> [w217]
    shift-right: [w212] -> _
    shift-left: FALSE -> [w211]
    stop <- w216 stop-if-true
    # "Pulse  Acquisition Loop"
    n61 = local read "Master Stop"() -> (w210:bool)
    n62 = case shown="False" w210 {
      tunnel: [w224 5122-States."Exit" ("Enum")] -> w214
      tunnel: w213 -> [w227 _]
      frame #0 {
        n63 = case shown="\"Standby\"" w227 {
          selector: w227 -> [w228 w229 w230 w231 w232 _]
          tunnel: [w228 w229 w230 w231 w232 5122-States."Initialize Card" ("Enum")] -> w226
          frame #0 {
          }
          frame #1 {
          }
          frame #2 {
          }
          frame #3 {
          }
          frame #4 {
          }
          frame #5 {
          }
        }
        n64 = Select(t=w226, s="Acquire Data", f=5122-States."Standby" ("Enum")) -> (s? t:f=w224:T10)
      }
      frame #1 {
      }
    }
    n65 = case shown="\"Fetch\"" w214 {
      selector: w214 -> [_ _ _ _ w400]
      tunnel: [w250 w288 w301 w398 w401] -> w222
      tunnel: [w248 w289 w295 w397 w402] -> w221
      tunnel: w220 -> [w253 w291 w300 w398 w401]
      tunnel: w219 -> [w252 w290 w299 w397 w402]
      tunnel: [5122-States."Continuous Mode" ("Enum") 5122-States."Fetch" ("Enum") w293 _ w400] -> w215
      tunnel: [_ _ _ TRUE ("Acquire Data") _] -> w216
      tunnel: [_ _ w296 _ _] -> w218
      tunnel: w217 -> [_ _ _ _ _]
      tunnel: [TRUE w286 _ _ _] -> w212
      tunnel: w211 -> [_ w286 w292 _ _]
      frame #0 {
        w235 = u8 0 ("Disabled")
        w262 = 0 items=["Positive", "Negative"] ("Trigger slope 6")
        w269 = TRUE  # Enforce realtime
        w259 = 1.0  # Probe attenuation
        w265 = u32 0 items=["1 mega ohm", "75 ohms", "50 ohms"]  # Input impedance
        # "Desired Number of Samples"
        n66 = property on="Capture" class="Bool"("Disabled"=w235) -> ()  [unwired: 2 in, 2 out]
        n67 = property on="Data Output" class="Path"("Disabled"=w235) -> ()  [unwired: 2 in, 2 out]
        n68 = property on="Total Acquired Time" class="DigNum (strict)"("Disabled"=w235) -> ()  [unwired: 2 in, 2 out]
        n69 = property on="Acquisition Sequence" class="WFGraph (strict)"("Disabled"=w235) -> ()  [unwired: 2 in, 2 out]
        n70 = property on="Total Experiment Time" class="DigNum (strict)"("Disabled"=w235) -> ()  [unwired: 2 in, 2 out]
        n71 = property on="Acquisitions Remaining" class="DigNum (strict)"("Disabled"=w235) -> ()  [unwired: 2 in, 2 out]
        n72 = property on="Number of Pulses to Record" class="DigNum (strict)"("Disabled"=w235) -> ()  [unwired: 2 in, 2 out]
        n73 = property on="Acquisition Time per Pulse" class="DigNum (strict)"("Disabled"=w235) -> ()  [unwired: 2 in, 2 out]
        n74 = property on="Channel" class="Ring (strict)"("Disabled"=w235) -> ()  [unwired: 2 in, 2 out]
        n75 = property on="Vertical coupling" class="Ring (strict)"("Disabled"=w235) -> ()  [unwired: 2 in, 2 out]
        n76 = property on="Vertical range (0 to 10V)" class="DigNum (strict)"("Disabled"=w235) -> ()  [unwired: 2 in, 2 out]
        n77 = property on="Desired Sample Rate" class="DigNum (strict)"("Disabled"=w235) -> ()  [unwired: 2 in, 2 out]
        n78 = property on="Acquisition Delay" class="DigNum (strict)"("Disabled"=w235) -> ()  [unwired: 2 in, 2 out]
        n79 = property on="Get Reference Parameters" class="Bool"("Disabled"=w235) -> ()  [unwired: 2 in, 2 out]
        n80 = disable-structure shown="Enabled" {
          frame #0 {
            w271 = 0
            n81 = property on="Falltime Chart" class="WFChart (strict)"("XScale.Minimum"=w271) -> ()  [unwired: 2 in, 2 out]
            n82 = property on="Width Chart" class="WFChart (strict)"("XScale.Minimum"=w271) -> ()  [unwired: 2 in, 2 out]
            n83 = property on="Risetime Chart" class="WFChart (strict)"("XScale.Minimum"=w271) -> ()  [unwired: 2 in, 2 out]
            n84 = property on="Amplitude Chart" class="WFChart (strict)"("XScale.RngStart"=w271) -> ()  [unwired: 2 in, 2 out]
            n85 = property on="Delay Chart" class="WFChart (strict)"("XScale.RngStart"=w271) -> ()  [unwired: 2 in, 2 out]
          }
          frame #1 {
          }
        }
        n86 = node("Vertical range (0 to 10V)") -> (w241:dbl)
        n87 = Number To Decimal String(number="Channel") -> (decimal integer string=w254:string)  [unwired: 1 out]
        "Channel String" <- w254
        n88 = node("Desired Sample Rate") -> (w246:dbl)
        n89 = local write "Acquisitions Remaining"(0 ("Acquisitions Remaining")) -> ()
        n90 = Multiply(x="Desired Sample Rate", y="Acquisition Time per Pulse") -> (x*y=w242:dbl)
        n91 = node(dbl[unit] 0.5 ("Trigger level")) -> (w256:dbl)
        n92 = case shown="1" "Vertical coupling" {
          tunnel: w241 -> [w276 w281 w284]
          tunnel: [0 0.0 w282] -> w238
          frame #0 {
            n93 = Divide(x=w276, y=2.0) -> (x/y=w274:dbl)
            n94 = Negate(x=w274) -> (-x=w273:dbl)
            n95 = property on="Acquisition Sequence" class="WFGraph (strict)"("YScale.Maximum"=w274, "YScale.Minimum"=w273) -> ()  [unwired: 2 in, 2 out]
          }
          frame #1 {
            n96 = Divide(x=w281, y=2.0) -> (x/y=w279:dbl)
            n97 = Negate(x=w279) -> (-x=w278:dbl)
            n98 = property on="Acquisition Sequence" class="WFGraph (strict)"("YScale.Maximum"=w279, "YScale.Minimum"=w278) -> ()  [unwired: 2 in, 2 out]
          }
          frame #2 {
            n99 = Divide(x=w284, y=2.0) -> (x/y=w282:dbl)
            n100 = property on="Acquisition Sequence" class="WFGraph (strict)"("YScale.Maximum"=w284, "YScale.Minimum"=0.0 ("Y Scale.Range:Minimum")) -> ()  [unwired: 2 in, 2 out]
          }
        }
        n101 = call <instrlib>:"niScope Configure Vertical.vi"("instrument handle"=w253, "probe attenuation"=w259, "vertical coupling"="Vertical coupling", "channels"=w254, "vertical range"=w241, "vertical offset"=w238, "error in"=w252) -> ("instrument handle out"=w268:refnum<k15>, "error out"=w267:errorcluster)  [unwired: 1 in, 6 out]
        n102 = call <instrlib>:"niScope Configure Chan Characteristics.vi"("instrument handle"=w268, "channels"=w254, "input impedance"=w265, "error in"=w267) -> ("instrument handle out"=w260:refnum<k15>, "error out"=w266:errorcluster)  [unwired: 1 in, 9 out]
        n103 = call <instrlib>:"niScope Configure Horizontal Timing.vi"("instrument handle"=w260, "enforce realtime"=w269, "min sample rate"=w246, "reference position"=0.0, "error in"=w266, "min record length"=w242) -> ("instrument handle out"=w263:refnum<k15>, "error out"=w264:errorcluster)  [unwired: 1 in, 7 out]
        n104 = node("Acquisition Delay") -> (w247:dbl)
        n105 = call-poly <instrlib>:"niScope Configure Trigger (poly).vi"("instrument handle"=w263, "trigger slope"=w262, "trigger source"="VAL_EXTERNAL" ("Trigger source"), "trigger level"=w256, "error in"=w264, "trigger delay"=w247) -> ("instrument handle out"=w251:refnum<k15>, "error out"=w249:errorcluster)  [unwired: 2 in, 6 out]
        n106 = call <instrlib>:"niScope Commit.vi"("instrument handle"=w251, "error in"=w249) -> ("instrument handle out"=w250:refnum<k15>, "error out"=w248:errorcluster)  [unwired: 12 out]
      }
      frame #1 {
        n107 = call <instrlib>:"niScope Initiate Acquisition.vi"("instrument handle"=w291, "error in"=w290) -> ("instrument handle out"=w288:refnum<k15>, "error out"=w289:errorcluster)  [unwired: 12 out]
      }
      frame #2 {
        # "clear file"
        n108 = call <instrlib>:"niScope Acquisition Status.vi"("instrument handle"=w300, "error in"=w299) -> ("instrument handle out"=w298:refnum<k15>, "acquisition status"=w294:i32, "error out"=w297:errorcluster)  [unwired: 11 out]
        n109 = case shown="0, Default" w294 {
          tunnel: [w304 w328] -> w301
          tunnel: w298 -> [w304 w373]
          tunnel: w297 -> [w303 w371]
          tunnel: [_ w306] -> w296
          tunnel: [5122-States."Fetch" ("Enum") w338] -> w293
          tunnel: [w303 w329] -> w295
          tunnel: w292 -> [_ _]
          frame #0 {
          }
          frame #1 {
            w355 = 1000.0 ("x")
            n110 = local read "Pulse Repetition Period"() -> (w326:dbl[unit])
            n111 = call <instrlib>:"niScope Actual Record Length.vi"("instrument handle"=w373, "error in"=w371) -> ("instrument handle out"=w372:refnum<k15>, "actual record length"=w327:i32, "error out"=w333:errorcluster)  [unwired: 11 out]
            "Number of Samples per Pulse" <- w327
            n112 = call <instrlib>:"niScope Sample Rate.vi"("instrument handle"=w372, "error in"=w333) -> ("instrument handle out"=w334:refnum<k15>, "actual sample rate"=w331:dbl, "error out"=w332:errorcluster)  [unwired: 11 out]
            n113 = local read "Acquisition Delay"() -> (w316:dbl[unit])
            n114 = node(w331) -> (w330:dbl[unit])
            "Actual Sample Rate" <- w330
            n115 = node(w326) -> (w341:dbl)
            n116 = property on="Risetime Chart" class="WFChart (strict)"("XScale.Multiplier"=w341) -> ("History Data"=w342:cluster{dbl}[])  [unwired: 2 in, 2 out]
            n117 = property on="Falltime Chart" class="WFChart (strict)"("XScale.Multiplier"=w341) -> ("History Data"=w347:cluster{dbl}[])  [unwired: 2 in, 2 out]
            n118 = property on="Width Chart" class="WFChart (strict)"("XScale.Multiplier"=w341) -> ("History Data"=w352:cluster{dbl}[])  [unwired: 2 in, 2 out]
            n119 = call "Timing Helper.vi"("Repetition Period"=w326, "Number of points per run"=w327, "Number of runs"="Number of Pulses to Record", "Sample rate"=w330) -> ("Total Experiment Time"=→"Total Experiment Time":dbl[unit], "Total Number of Datapoints"=→"Total Number of Datapoints":i64, "Total Acquired Time"=→"Total Acquired Time":dbl[unit], "Acquisition Time per Run"=w311:dbl[unit])
            n120 = property on="Delay Chart" class="WFChart (strict)"("XScale.Multiplier"=w341) -> ("History Data"=w353:cluster{dbl}[])  [unwired: 2 in, 2 out]
            n121 = property on="Amplitude Chart" class="WFChart (strict)"("XScale.Multiplier"=w341) -> ("History Data"=w354:cluster{dbl}[])  [unwired: 2 in, 2 out]
            n122 = Add(x=w316, y=w311) -> (x+y=w315:dbl[unit])
            n123 = node(w316) -> (w319:dbl)
            n124 = node(w315) -> (w318:dbl)
            n125 = local read "Channel String"() -> (w336:string)
            n126 = call "Stats Formatter.vi"("Unit String"=" ns" ("string"), "History Data"=w342, "factor"=w355) -> ("Statistics String"=→"Risetime":string)  [unwired: 2 out]
            n127 = call "Stats Formatter.vi"("Unit String"=" ns" ("string"), "History Data"=w347, "factor"=w355) -> ("Statistics String"=→"Falltime":string)  [unwired: 2 out]
            n128 = call "Stats Formatter.vi"("History Data"=w352) -> ("Statistics String"=→"Pulse Width":string)  [unwired: 2 in, 2 out]
            n129 = call "Stats Formatter.vi"("History Data"=w353) -> ("Statistics String"=→"Delay":string, "Mean"=w320:dbl)  [unwired: 2 in, 1 out]
            n130 = call "Stats Formatter.vi"("Unit String"=" V" ("string"), "History Data"=w354) -> ("Statistics String"=→"Amplitude":string)  [unwired: 1 in, 2 out]
            n131 = property on="Acquisition Sequence" class="WFGraph (strict)"("XScale.Offset"=w319, "XScale.Minimum"=w319, "XScale.ScaleFit"=u8 0 ("X Scale.Scale Fit"), "XScale.Maximum"=w318) -> ()  [unwired: 2 in, 2 out]
            n132 = call-poly <instrlib>:"niScope Fetch (poly).vi"("timeout"=0.0, "error in"=w332, "channels"=w336, "instrument handle"=w334) -> ("error out"=w329:errorcluster, "wfm"=w306:dbl[], "instrument handle out"=w328:refnum<k15>)  [unwired: 1 in, 4 out]
            n133 = event shown="[1] \"Capture\": Value Change" {
              selector: _ -> [_ _ _ _]
              dyn-events: _ -> [_ _ _ _]
              timeout: 0 -> [_ _ _ _]
              tunnel: [5122-States."Continuous Mode" ("Enum") 5122-States."Continuous Mode" ("Enum") 5122-States."Initialize Card" ("Enum") 5122-States."Continuous Mode" ("Enum")] -> w324
              tunnel: w306 -> [_ _ _ w388]
              event #0 {
                n134 = event-data() -> ()  [unwired: 3 out]
              }
              event #1 {
                # "clear file"
                n135 = event-data() -> ()  [unwired: 2 out]
                n136 = call-poly <vilib>:"Write To Spreadsheet File.vi"("file path (dialog if empty)"="Data Output") -> ()  [unwired: 5 in, 3 out]
                n137 = local read "Number of Pulses to Record"() -> (→"Acquisitions Remaining":i32)
              }
              event #2 {
                n138 = event-data() -> ()  [unwired: 3 out]
              }
              event #3 {
                n139 = event-data() -> ()  [unwired: 5 out]
                n140 = local read "Data Output"() -> (w394:path)
                n141 = Strip Path(path=w394) -> (stripped path=w395:path)  [unwired: 1 out]
                n142 = Build Path(base path=w395, name or relative path="reference-pulse.txt") -> (appended path=w392:path)
                n143 = call-poly <vilib>:"Write To Spreadsheet File.vi"("transpose? (no:F)"=TRUE ("append to file? (new file:F)"), "format (%.3f)"="%.7f", "1D data"=w388, "file path (dialog if empty)"=w392) -> ()  [unwired: 2 in, 3 out]
                "Reference Pulse" <- w388
              }
            }
            n144 = local read "Actual Sample Rate"() -> (w325:dbl[unit])
            n145 = local read "Reference Pulse"() -> (w307:dbl[])
            n146 = local read "Acquisitions Remaining"() -> (w308:i32)
            n147 = Reciprocal(x=w325) -> (1/x=w369:dbl[unit])
            "Interval Between Samples" <- w369
            n148 = call <vilib>:"Pulse Parameters.vi"("X"=w306) -> ("risetime"=w359:dbl, "amplitude"=w322:dbl, "delay"=w356:dbl, "duration"=w357:dbl, "falltime"=w358:dbl)  [unwired: 10 out]
            n149 = node(w369) -> (w370:dbl)
            n150 = Build Array(w306, w307) -> (→"Acquisition Sequence":dbl[][])
            n151 = Greater Than 0?(x=w308) -> (x > 0?=w309:bool)
            n152 = property on="Acquisition Sequence" class="WFGraph (strict)"("XScale.Multiplier"=w370) -> ()  [unwired: 2 in, 2 out]
            n153 = Multiply(x=w370, y=w357) -> (x*y=w367:dbl)
            n154 = Multiply(x=w370, y=w356) -> (x*y=w368:dbl)
            n155 = Multiply(x=w370, y=w358) -> (x*y=w366:dbl)
            n156 = Multiply(x=w370, y=w359) -> (x*y=w360:dbl)
            n157 = case shown="True" w309 {
              tunnel: w306 -> [_ w380]
              tunnel: [_ TRUE ("Blinking")] -> w323
              tunnel: w308 -> [_ w377]
              frame #0 {
              }
              frame #1 {
                w381 = TRUE ("append to file? (new file:F)")
                n158 = local read "Data Output"() -> (w376:path)
                n159 = Decrement(x=w377) -> (x-1=w379:i32)
                n160 = local write "Acquisitions Remaining"(w379) -> ()
                n161 = call-poly <vilib>:"Write To Spreadsheet File.vi"("transpose? (no:F)"=w381, "format (%.3f)"="%.7f", "append to file? (new file:F)"=w381, "1D data"=w380, "file path (dialog if empty)"=w376) -> ()  [unwired: 1 in, 3 out]
              }
            }
            n162 = Less Than 0?(x=w322) -> (x < 0?=w321:bool)
            n163 = Bundle(w360) -> (→"Risetime Chart":cluster{dbl})  [unwired: 1 in]
            n164 = Bundle(w366) -> (→"Falltime Chart":cluster{dbl})  [unwired: 1 in]
            n165 = Bundle(w367) -> (→"Width Chart":cluster{dbl})  [unwired: 1 in]
            n166 = Bundle(w368) -> (→"Delay Chart":cluster{dbl})  [unwired: 1 in]
            n167 = Bundle("amplitude"=w322) -> (→"Amplitude Chart":cluster{"amplitude":dbl})  [unwired: 1 in]
            n168 = case shown="False" w321 {
              tunnel: w320 -> [_ w375]
              frame #0 {
              }
              frame #1 {
                # "Time needed to add to EIT \nsignal delay since pulse doesn't start \nright when we recieve trigger"
                n169 = node(w375) -> (→"Global EIT Delay":dbl[unit])
              }
            }
            n170 = Unbundle By Name(w329) -> ("status"=w339:bool)
            n171 = property on="Acquire Data" class="Bool (strict)"("Blinking"=w323) -> ()  [unwired: 2 in, 2 out]
            n172 = Select(t=5122-States."Exit" ("Enum"), s=w339, f=w324) -> (s? t:f=w338:T10)
          }
        }
      }
      frame #3 {
      }
      frame #4 {
        w399 = u8 2 ("Disabled")
        n173 = property on="Acquisition Time per Pulse" class="DigNum (strict)"("Disabled"=w399) -> ()  [unwired: 2 in, 2 out]
        n174 = property on="Capture" class="Bool"("Disabled"=w399) -> ()  [unwired: 2 in, 2 out]
        n175 = property on="Data Output" class="Path"("Disabled"=w399) -> ()  [unwired: 2 in, 2 out]
        n176 = property on="Total Acquired Time" class="DigNum (strict)"("Disabled"=w399) -> ()  [unwired: 2 in, 2 out]
        n177 = property on="Acquisition Sequence" class="WFGraph (strict)"("Disabled"=w399) -> ()  [unwired: 2 in, 2 out]
        n178 = property on="Total Experiment Time" class="DigNum (strict)"("Disabled"=w399) -> ()  [unwired: 2 in, 2 out]
        n179 = property on="Number of Pulses to Record" class="DigNum (strict)"("Disabled"=w399) -> ()  [unwired: 2 in, 2 out]
        n180 = property on="Channel" class="Ring (strict)"("Disabled"=w399) -> ()  [unwired: 2 in, 2 out]
        n181 = property on="Vertical coupling" class="Ring (strict)"("Disabled"=w399) -> ()  [unwired: 2 in, 2 out]
        n182 = property on="Vertical range (0 to 10V)" class="DigNum (strict)"("Disabled"=w399) -> ()  [unwired: 2 in, 2 out]
        n183 = property on="Desired Sample Rate" class="DigNum (strict)"("Disabled"=w399) -> ()  [unwired: 2 in, 2 out]
        n184 = property on="Acquisition Delay" class="DigNum (strict)"("Disabled"=w399) -> ()  [unwired: 2 in, 2 out]
        n185 = property on="Acquisitions Remaining" class="DigNum (strict)"("Disabled"=w399) -> ()  [unwired: 2 in, 2 out]
        n186 = property on="Get Reference Parameters" class="Bool"("Disabled"=w399) -> ()  [unwired: 2 in, 2 out]
      }
    }
  }
  n187 = while {
    shift-right: [w404] -> _
    shift-left: States."Initialize" ("Enum") -> [w410]
    tunnel: w17 -> [w409]
    tunnel: w15 -> [w408]
    tunnel: [w407] -> w20
    tunnel: [w406] -> w19
    stop <- w403 stop-if-true
    n188 = case shown="\"Receive Data\"" w410 {
      selector: w410 -> [_ _ _ w488 _ _]
      tunnel: w409 -> [w415 w459 w478 w493 w567 w586]
      tunnel: w408 -> [w412 w458 w477 w486 w566 w585]
      tunnel: [w413 w455 w478 w492 w568 w586] -> w407
      tunnel: [w411 w453 w477 w491 w561 w585] -> w406
      tunnel: [_ _ _ w490 _ _] -> w403
      tunnel: [States."Send Data" ("Enum") States."Check for Activity" ("Enum") w472 w488 w557 States."Check for Activity" ("Enum")] -> w404
      frame #0 {
        n189 = disable-structure shown="Enabled" {
          disable-tunnel: w415 -> [w421 w423]
          disable-tunnel: [w420 w423] -> w413
          disable-tunnel: w412 -> [w418 w422]
          disable-tunnel: [w417 w422] -> w411
          frame #0 {
            n190 = xnode "Invoke Method"("FPGA VI Reference In"=w421, "error in"=w418, "Depth"=u32 400000) -> ("FPGA VI Reference Out"=w420:refnum<k20>, "error out"=w417:errorcluster)
          }
          frame #1 {
          }
        }
        n191 = property on="Active" class="Bool (strict)"("Blinking"=TRUE) -> ()  [unwired: 2 in, 2 out]
      }
      frame #1 {
        n192 = xnode "Read/Write Control"("FPGA VI Reference In"=w459, "error in"=w458) -> ("FPGA VI Reference Out"=w456:refnum<k20>, "error out"=w454:errorcluster, "Last Chopper Period"=w444:u64, "Last Global Period"=w445:u64, "Last Memory Period"=w442:u64, "Last DLCZ Period"=w441:u64, "T_last-chop + t_dark"=w440:u64, "t_last_chop+t_dark-t_off"=w425:u64, "t_chop"=w439:u64, "Global Time"=w438:u64, "Memory Timer"=w437:u64, "Memory Mode"=→"Memory Mode 2":T3, "Time to Cut B"=w428:u64, "Current State"=→"Current State":T5)
        n193 = call "Convert Ticks to Time.vi"("Ticks"=w445) -> ("Time"=→"Acquisition Rate":dbl[unit])
        n194 = call "Convert Ticks to Time.vi"("Ticks"=w442) -> ("Time"=→"Memory Sequence Duration":dbl[unit])
        n195 = call "Convert Ticks to Time.vi"("Ticks"=w441) -> ("Time"=→"Last DLCZ Period":dbl[unit])
        n196 = call "Convert Ticks to Time.vi"("Ticks"=w440) -> ("Time"=→"T_last-chop + t_dark":dbl[unit])
        n197 = call "Convert Ticks to Time.vi"("Ticks"=w439) -> ("Time"=→"t_chop":dbl[unit])
        n198 = call "Convert Ticks to Time.vi"("Ticks"=w438) -> ("Time"=→"Global Time":dbl[unit])
        n199 = call "Convert Ticks to Time.vi"("Ticks"=w437) -> ("Time"=→"Memory Timer":dbl[unit])
        n200 = call "Convert Ticks to Time.vi"("Ticks"=w428) -> ("Time"=→"B-Field Extinction Time 2":dbl[unit])
        n201 = call "Convert Ticks to Time.vi"("Ticks"=w425) -> ("Time"=→"t_last_chop+t_dark-t_off":dbl[unit])
        n202 = call "Convert Ticks to Time.vi"() -> ()  [unwired: 1 in, 1 out]
        n203 = call "Convert Ticks to Time.vi"("Ticks"=w444) -> ("Time"=w443:dbl[unit])
        n204 = local write "Pulse Repetition Period"(w443) -> ()
        n205 = Divide(x=6.25, y=360) -> (x/y=w452:dbl)
        n206 = Multiply(x=w444, y=w452) -> (x*y=w449:dbl)
        n207 = Round To Nearest(number=w449) -> (nearest integer value=w448:dbl)
        n208 = To Unsigned Quad Integer(1:w448) -> (0:w447:u64)
        n209 = call "Convert Ticks to Time.vi"("Ticks"=w447) -> ("Time"=→"Chopper 1/2 Dark Time":dbl[unit])  [unwired: 19 in, 7 out]
        n210 = xnode "Read/Write Control"("FPGA VI Reference In"=w456, "error in"=w454, "Chopper Dark Time"=w447) -> ("FPGA VI Reference Out"=w455:refnum<k20>, "error out"=w453:errorcluster)
      }
      frame #2 {
        n211 = event shown="[1] \"Control Duration (DIO5/1) \", \"Pump (DIO8) \", \"Repump (DIO4)\", \"Signal Delay (DIO6)\", \"Signal Duration (DIO6)\", \" Signal Trigger Source (DIO0)\", \"Pulse Selection\", \"Switch Chopper \nWindow Trigger\", \"Output  Trigger Sign (DIO1)\", \"DLCZ Pulse Duration\", \" DLCZ Period\", \"Opt Density Duration (DIO7)\", \"Opt Density Delay (DIO7)\", \"Trapping (DIO3)\", \"Memory Mode\", \"Control Delay(DIO5/1)\", \"Min. Measurement Period\", \"B-Field Extinction Time\", \"Epsilon\", \" DLCZ Start\", \" DLCZ Stop\", \"A\", \"B\", \"Global Delay\", \"Raman Signal Duration (DIO6)\", \"Raman Signal Delay (DIO6)\", \"Raman Control Delay(DIO5)\", \"Ramand Control Duration (DIO5) \": Value Change;  \"Pulse Repetition Period\": Key Down" {
          selector: _ -> [_ _ _]
          dyn-events: _ -> [_ _ _]
          timeout: 100 -> [_ _ _]
          tunnel: [w479 States."Send Data" ("Enum") States."Close" ("Enum")] -> w473
          event #0 {
            n212 = event-data() -> ()  [unwired: 3 out]
            n213 = local read "Signal Trigger Source (DIO0)"() -> (w482:bool)
            n214 = Select(t=States."Update Graph" ("Enum"), s=w482, f=States."Receive Data" ("Enum")) -> (s? t:f=w479:T7)
          }
          event #1 {
            n215 = event-data() -> ()  [unwired: 5 out]
          }
          event #2 {
            n216 = event-data() -> ()  [unwired: 4 out]
          }
        }
        n217 = local read "Master Stop"() -> (w475:bool)
        n218 = Select(t=States."Close" ("Enum"), s=w475, f=w473) -> (s? t:f=w472:T7)
      }
      frame #3 {
        w490 = TRUE ("Stop")
        n219 = disable-structure shown="Enabled" {
          disable-tunnel: w493 -> [w497 w499]
          disable-tunnel: [w496 w499] -> w487
          disable-tunnel: w486 -> [w495 w498]
          disable-tunnel: [w494 w498] -> w485
          frame #0 {
            n220 = xnode "Invoke Method"("FPGA VI Reference In"=w497, "error in"=w495) -> ("FPGA VI Reference Out"=w496:refnum<k20>, "error out"=w494:errorcluster)
          }
          frame #1 {
          }
        }
        n221 = xnode "Read/Write Control"("FPGA VI Reference In"=w487, "error in"=w485, "Stop"=w490) -> ("FPGA VI Reference Out"=w492:refnum<k20>, "error out"=w491:errorcluster)
        "Active" <- FALSE ("Active 2")
      }
      frame #4 {
        w506 = FALSE ("Show Errors")
        w516 = FALSE ("Show Errors")
        w525 = FALSE ("Show Errors")
        w518 = FALSE ("Show Errors")
        w515 = 40
        # "Chopper Decimation and EIT Sequence Loop"
        n222 = local read "Memory Duration"() -> (w543:dbl[unit])
        n223 = local read "Cut Initiated"() -> (w517:dbl[unit])
        n224 = call "HostConvertTimetoTicks.vi"("Clock Factor"=w515, "Duration (us)"="Min. Measurement Period", "Show Errors"=w525) -> ("duration (tick numbers)"=w544:u64)  [unwired: 9 in, 3 out]
        n225 = call "HostConvertTimetoTicks.vi"("Clock Factor"=w515, "Duration (us)"="B-Field Extinction Time", "Show Errors"=FALSE) -> ("duration (tick numbers)"=w541:u64)  [unwired: 9 in, 3 out]
        n226 = call "HostConvertTimetoTicks.vi"("Clock Factor"=w515, "Duration (us)"=w543, "Show Errors"=FALSE) -> ("duration (tick numbers)"=w545:u64)  [unwired: 9 in, 3 out]
        n227 = call "HostConvertTimetoTicks.vi"("Clock Factor"=w515, "Duration (us)"=w517, "Show Errors"=w516) -> ()  [unwired: 9 in, 4 out]
        n228 = call "HostConvertTimetoTicks.vi"("Clock Factor"=w515, "Duration (us)"="DLCZ Start", "Show Errors"=w525) -> ("duration (tick numbers)"=w524:u64)  [unwired: 9 in, 3 out]
        n229 = call "HostConvertTimetoTicks.vi"("Repetition Period"="DLCZ Period", "Clock Factor"=w515, "Duration (us)"="DLCZ Pulse Duration", "Show Errors"=w518) -> ("duration (tick numbers)"=w533:u64)  [unwired: 8 in, 3 out]
        n230 = call "HostConvertTimetoTicks.vi"("Clock Factor"=w515, "Duration (us)"="DLCZ Period", "Show Errors"=w518) -> ("duration (tick numbers)"=w519:u64)  [unwired: 9 in, 3 out]
        n231 = call "Scale Frequency.vi"("Period"="Pulse Repetition Period") -> ("Frequency (scaled)"=w563:u32)
        n232 = call "HostConvertTimetoTicks.vi"("Repetition Period"="Pulse Repetition Period", "Clock Factor"=w515, "Delay (us)"="Control Delay(DIO5/1)", "Duration (us)"="Control Duration (DIO5/1)") -> ("start pulse (tick number)"=w575:u64, "stop pulse (tick number)"=w574:u64)  [unwired: 8 in, 2 out]
        n233 = call "HostConvertTimetoTicks.vi"("Repetition Period"="Pulse Repetition Period", "Clock Factor"=w515, "Duration (us)"="Trapping (DIO3)", "Show Errors"=FALSE) -> ("duration (tick numbers)"=w537:u64)  [unwired: 8 in, 3 out]
        n234 = call "HostConvertTimetoTicks.vi"("Repetition Period"="Pulse Repetition Period", "Clock Factor"=w515, "Duration (us)"="Pump (DIO8)", "Show Errors"=FALSE) -> ("duration (tick numbers)"=w536:u64)  [unwired: 8 in, 3 out]
        n235 = call "HostConvertTimetoTicks.vi"("Repetition Period"="Pulse Repetition Period", "Clock Factor"=w515, "Duration (us)"="Repump (DIO4)") -> ("duration (tick numbers)"=w538:u64)  [unwired: 9 in, 3 out]
        n236 = call "HostConvertTimetoTicks.vi"("Repetition Period"="Pulse Repetition Period", "Clock Factor"=w515, "Delay (us)"="Signal Delay (DIO6)", "Duration (us)"="Signal Duration (DIO6)") -> ("start pulse (tick number)"=w549:u64, "stop pulse (tick number)"=w548:u64)  [unwired: 8 in, 2 out]
        n237 = call "HostConvertTimetoTicks.vi"("Repetition Period"="Pulse Repetition Period", "Clock Factor"=w515, "Delay (us)"="Opt Density Delay (DIO7)", "Duration (us)"="Opt Density Duration (DIO7)") -> ("start pulse (tick number)"=w535:u64, "stop pulse (tick number)"=w534:u64)  [unwired: 8 in, 2 out]
        n238 = call "HostConvertTimetoTicks.vi"("Clock Factor"=w515, "Duration (us)"="DLCZ Stop", "Show Errors"=FALSE) -> ("duration (tick numbers)"=w522:u64)  [unwired: 9 in, 3 out]
        n239 = call "HostConvertTimetoTicks.vi"("Clock Factor"=w515, "Delay (us)"="Raman Control Delay(DIO5)", "Duration (us)"="Ramand Control Duration (DIO5)", "Show Errors"=w506) -> ("start pulse (tick number)"=w510:u64, "stop pulse (tick number)"=w509:u64)  [unwired: 8 in, 2 out]
        n240 = call "HostConvertTimetoTicks.vi"("Clock Factor"=w515, "Delay (us)"="Raman Signal Delay (DIO6)", "Duration (us)"="Raman Signal Duration (DIO6)", "Show Errors"=w506) -> ("start pulse (tick number)"=w512:u64, "stop pulse (tick number)"=w511:u64)  [unwired: 8 in, 2 out]
        n241 = call "HostConvertTimetoTicks.vi"("Clock Factor"=w515, "Duration (us)"="Epsilon", "Show Errors"=w516) -> ("duration (tick numbers)"=w527:u64)  [unwired: 9 in, 3 out]
        n242 = xnode "Read/Write Control"("FPGA VI Reference In"=w567, "error in"=w566, "Control - start"=w575, "Control - stop"=w574, "Signal start"=w549, "Signal stop"=w548, "Trapping Duration"=w537, "Pump Duration"=w536, "Repump Duration"=w538, "Optical Density - start"=w535, "Optical Density - stop"=w534, "Repetition Period"=w563, "DLCZ width"=w533, "DLCZ Period"=w519, "DLCZ Start"=w524, "DLCZ Stop"=w522, "Pulse Selection"="Pulse Selection", "Switch Trigger (Shift Decimation)"="Switch Chopper \nWindow Trigger", "Trigger Source"="Signal Trigger Source (DIO0)", "Output Trigger Sign"="Output  Trigger Sign (DIO1)", "Minimum Period Between Memory Sequences"=w544, "Time to Cut B"=w541, "Memory Sequence Duration"=w545, "Memory Mode"="Memory Mode", "epsilon"=w527, "Raman Control - start"=w510, "Raman Control - stop"=w509, "Raman Signal - start"=w512, "Raman Signal - stop"=w511) -> ("FPGA VI Reference Out"=w568:refnum<k20>, "error out"=w561:errorcluster)
        n243 = Unbundle By Name(w561) -> ("status"=w562:bool)
        n244 = Compound Arithmetic op=OR(w562, "Master Stop") -> (w556:bool)
        n245 = case shown="False" "Signal Trigger Source (DIO0)" {
          frame #0 {
            n246 = property on="Pulse Repetition Period" class="DigNum (strict)"("Disabled"=u8 2) -> ()  [unwired: 2 in, 2 out]
          }
          frame #1 {
            n247 = local write "Pulse Selection"(FALSE) -> ()
            n248 = property on="Pulse Repetition Period" class="DigNum (strict)"("Disabled"=u8 0) -> ()  [unwired: 2 in, 2 out]
          }
        }
        n249 = Select(t=States."Close" ("Enum"), s=w556, f=States."Update Graph" ("Enum")) -> (s? t:f=w557:T7)
      }
      frame #5 {
        n250 = feedback #1() -> (w587:bool)  [unwired: 1 out]
        "Graphing" <- w587
        n251 = Not(x=w587) -> (.not. x?=w588:bool)
      }
    }
    n252 = Wait (ms)(milliseconds to wait=u32 100) -> ()  [unwired: 1 out]
  }
  n253 = while {
    shift-right: [w593] -> _
    shift-left: B-Generator_States."Initialize" ("B-Generator States") -> [w594]
    shift-right: [w595] -> w30
    shift-left: errorcluster {"status"=FALSE, "code"=0, "source"=""} ("error out") -> [w590]
    shift-right: [w596] -> w31
    shift-left: _ -> [w591]
    stop <- w592 stop-if-true
    # "B Field Control Signal Generator"
    n254 = case shown="\"Initialize\"" w594 {
      tunnel: [w632 w644 w651 w673 w677] -> w596
      tunnel: [w631 w645 w650 w672 w676] -> w595
      tunnel: [B-Generator_States."Start Task" ("B-Generator States") B-Generator_States."Check Task" ("B-Generator States") w649 B-Generator_States."Start Task" ("B-Generator States") B-Generator_States."Stop" ("B-Generator States")] -> w593
      tunnel: [_ _ _ _ TRUE] -> w592
      tunnel: w591 -> [w630 w647 w653 w675 w677]
      tunnel: w590 -> [w635 w646 w652 w674 w676]
      frame #0 {
        w602 = 10171 items=["Rising"=10280, "Falling"=10171] ("edge")
        w613 = 250000.0
        w642 = 10178 items=["Finite Samples"=10178, "Continuous Samples"=10123] ("sample mode")
        # "Write Waveform to\nhardware buffer"
        # "Output Pin"
        # "Start Generation on a trigger \nfrom this pin"
        # "Needed so it only writes \nwaveform once per trigger"
        n255 = call-poly <vilib>:"DAQmx Create Virtual Channel.vi"("task in"=w630, "physical channels"=tag "Julien/ao0" ("Physical Channels"), "error in"=w635) -> ("task out"=w637:refnum<k21>, "error out"=w636:errorcluster)  [unwired: 7 in, 4 out]
        n256 = Select(t="High Voltage (V Hi)", s="Activate B-Field", f=dbl[unit] 0.0 ("Ground")) -> (s? t:f=w608:dbl[unit])
        n257 = call "B-Field Array Generator.vi"("Final Voltage"="V2", "Initial Voltage"="V1", "Time"="A", "Sample Rate"=w613) -> ("Voltage Ouputs"=w633:dbl[])
        n258 = call "B-Field Array Generator.vi"("Final Voltage"="V4", "Initial Voltage"="V3", "Time"="B", "Sample Rate"=w613) -> ("Voltage Ouputs"=w634:dbl[])
        n259 = call "B-Field Array Generator.vi"("Final Voltage"=w608, "Initial Voltage"=w608, "Time"="Global Delay", "Sample Rate"=w613) -> ("Voltage Ouputs"=w612:dbl[])
        n260 = Add(x="Global Delay", y="A") -> (x+y=→"Cut Initiated":dbl[unit])
        n261 = Compound Arithmetic op=ADD("A", "B") -> (→"Memory Duration":dbl[unit])
        n262 = local read "Activate B-Field"() -> (w604:bool)
        n263 = call-poly <vilib>:"DAQmx Timing.vi"("task/channels in"=w637, "sample mode"=w642, "rate"=w613, "error in"=w636) -> ("task out"=w625:refnum<k21>, "error out"=w640:errorcluster)  [unwired: 3 in, 7 out]
        n264 = Build Array (concatenate)(w633, w634) -> (w611:dbl[])
        n265 = Build Array (concatenate)(w612, w611, w612) -> (w614:dbl[])
        n266 = And(x="Trigger Control", y=w604) -> (x .and. y?=w605:bool)
        n267 = Select(t=w614, s=w605, f=w612) -> (s? t:f=w606:dbl[])
        n268 = call-poly <vilib>:"DAQmx Trigger.vi"("task/channels in"=w625, "source"=tag "/Julien/PFI0" ("Trigger Source"), "edge"=w602, "error in"=w640) -> ("task out"=w624:refnum<k21>, "error out"=w623:errorcluster)  [unwired: 10 out]
        n269 = Reciprocal(x=w613) -> (1/x=w628:dbl)
        n270 = call "B-Field - Bug1 Workaround.vi"("Array 2"=w606) -> ("Array"=w610:dbl[])
        "B-Field Control Signal" <- w610
        n271 = Multiply(x=w628, y=1000.0) -> (x*y=w627:dbl)
        n272 = Array Size(array=w610) -> (size(s)=w620:i32)
        n273 = property class="DAQmx Timing"(reference=w624, error in=w623, "SampQuant.SampPerChan"=w620) -> (reference out=w622:refnum<k21>, error out=w621:errorcluster)
        n274 = Multiply(x=w627, y=w620) -> (x*y=w626:dbl)
        n275 = property on="B-Field Control Signal" class="WFGraph (strict)"("XScale.Multiplier"=w627, "XScale.Maximum"=w626) -> ()  [unwired: 2 in, 2 out]
        n276 = call-poly <vilib>:"DAQmx Write.vi"("task/channels in"=w622, "data"=w610, "error in"=w621) -> ("task out"=w632:refnum<k21>, "error out"=w631:errorcluster)  [unwired: 1 in, 10 out]
      }
      frame #1 {
        n277 = call <vilib>:"DAQmx Start Task.vi"("task/channels in"=w647, "error in"=w646) -> ("task out"=w644:refnum<k21>, "error out"=w645:errorcluster)  [unwired: 12 out]
      }
      frame #2 {
        n278 = event shown="[0] Timeout" {
          selector: _ -> [_ _]
          dyn-events: _ -> [_ _]
          timeout: 0 -> [_ _]
          tunnel: [w661 B-Generator_States."Initialize" ("B-Generator States")] -> w654
          tunnel: [w659 _] -> w651
          tunnel: w653 -> [w666 w669]
          tunnel: w652 -> [w665 w668]
          tunnel: [w660 w667] -> w650
          event #0 {
            n279 = event-data() -> ()  [unwired: 2 out]
            n280 = call <vilib>:"DAQmx Is Task Done.vi"("task/channels in"=w666, "error in"=w665) -> ("task out"=w659:refnum<k21>, "task done?"=w664:bool, "error out"=w660:errorcluster)  [unwired: 1 in, 10 out]
            n281 = Select(t=B-Generator_States."Stop Task" ("B-Generator States"), s=w664, f=B-Generator_States."Check Task" ("B-Generator States")) -> (s? t:f=w661:T9)
          }
          event #1 {
            n282 = event-data() -> ()  [unwired: 7 out]
            n283 = call <vilib>:"DAQmx Clear Task.vi"("task in"=w669, "error in"=w668) -> ("error out"=w667:errorcluster)  [unwired: 13 out]
          }
        }
        n284 = local read "Master Stop"() -> (w648:bool)
        n285 = Unbundle By Name(w650) -> ("status"=w658:bool)
        n286 = Or(x=w658, y=w648) -> (x .or. y?=w657:bool)
        n287 = Select(t=B-Generator_States."Stop" ("B-Generator States"), s=w657, f=w654) -> (s? t:f=w649:T9)
      }
      frame #3 {
        n288 = call <vilib>:"DAQmx Stop Task.vi"("task/channels in"=w675, "error in"=w674) -> ("task out"=w673:refnum<k21>, "error out"=w672:errorcluster)  [unwired: 12 out]
      }
      frame #4 {
      }
    }
  }
  n289 = call <vilib>:"DAQmx Clear Task.vi"("task in"=w31, "error in"=w30) -> ("error out"=w32:errorcluster)  [unwired: 13 out]
  n290 = call <vilib>:"Simple Error Handler.vi"("type of dialog (OK msg:1)"=w33, "error in (no error)"=w32) -> ("error out"=w27:errorcluster)  [unwired: 7 out]
  n291 = xnode "Close FPGA VI Reference"("FPGA VI Reference In"=w20, "error in"=w19) -> ("error out"=w21:errorcluster)
  n292 = call <instrlib>:"RF On_OFF.vi"("VISA Resource Name"=w14, "error in (no error)"=w6) -> ("VISA Resource Name Out"=w10:refnum<visa-resource-name>, "error out"=w9:errorcluster)  [unwired: 1 in, 11 out]
  n293 = call <instrlib>:"Error Query.vi"("VISA Resource Name"=w10, "error in (no error)"=w9) -> ("VISA Resource Name Out"=w11:refnum<visa-resource-name>, "error out"=w8:errorcluster)  [unwired: 12 out]
  n294 = call <vilib>:"Simple Error Handler.vi"("error in (no error)"=w21) -> ("error out"=w26:errorcluster)  [unwired: 1 in, 7 out]
  n295 = call <instrlib>:"Error Message.vi"("VISA Resource Name"=w11, "error in (no error)"=w8) -> ("VISA Resource Name Out"=w12:refnum<visa-resource-name>, "error out"=w7:errorcluster)  [unwired: 1 in, 11 out]
  n296 = property on="Acquire Data" class="Bool (strict)"(error in=w43, "Value"=FALSE ("Acquire Data")) -> (error out=w42:errorcluster)  [unwired: 1 in, 1 out]
  n297 = call <instrlib>:"Close.vi"("VISA Resource Name"=w12, "error in (no error)"=w7) -> ()  [unwired: 14 out]
  n298 = call <instrlib>:"niScope Close.vi"("instrument handle"=w50, "error in"=w42) -> ("error out"=w51:errorcluster)  [unwired: 13 out]
  n299 = call <vilib>:"Simple Error Handler.vi"("error in (no error)"=w51) -> ("error out"=w25:errorcluster)  [unwired: 1 in, 7 out]
  n300 = call <vilib>:"Merge Errors.vi"("error in 3 (no error)"=w25, "error in 2 (no error)"=w26, "error in 1 (no error)"=w27) -> ("error out"=w23:errorcluster)  [unwired: 1 in, 3 out]
  n301 = case shown="True" TRUE {
    tunnel: w23 -> [w680 w682]
    tunnel: [w680 w682] -> w22
    frame #0 {
    }
    frame #1 {
      n302 = local write "Master Stop"(FALSE ("Master Stop")) -> ()
    }
  }
  n303 = disable-structure shown="Disabled" {
    disable-tunnel: w22 -> [w683 _]
    frame #0 {
      n304 = invoke class="VI" method="Default Vals.Reinit All"(error in=w683) -> ()  [unwired: 2 in, 3 out]
    }
    frame #1 {
    }
  }
